vi "Image.vi"(8 "error in":errorcluster) -> (0 "error out":errorcluster)   [LabVIEW 2019, in "Image.lvlib"]
uses:
  Image.lvlib
  User Event/Controls/UE Abort Action.ctl
  LED/SubVI/Image Para.ctl
  MiControl-E/LV Source/ImageSystem/Cradle Zyla_1117/Ctl/seletion.ctl
  <vilib>/vision/Image Controls.llb/IMAQ Image.ctl
  <vilib>/Utility/error.llb/Error Cluster From Error Code.vi
  <vilib>/ErrorRing/Error Ring.xnode
  Queues/Queues.lvlib
  LED/LED.lvlib
  Motion/Allmotion/Allmotion.lvlib
  Camera/Andor/Andor.lvlib
  <vilib>/vision/NI_Vision_Development_Module.lvlib
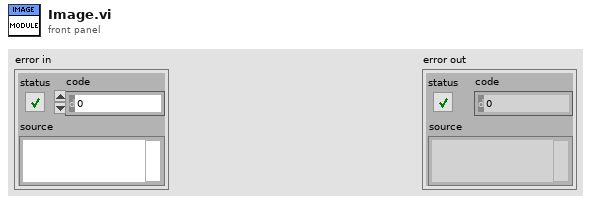
[diagram p1: front panel]
types:
  T1 = typedef "LED.lvlib/Image Para.ctl" = cluster{"Marker":T2, "Power(Amp)":u8, "set shutter(s)":dbl, "Cube":enum16{"1", "2", "3", "4", "5", "6", "7", "8"}}
  T2 = typedef "seletion.ctl" = enum16{"None", "Red", "Green", "Blue", "UV", "Green Laser", "Blue-Red", "UV-Red", "BF", "UV-IR"}
  T3 = typedef "IMAQ Image.ctl" = refnum<image>
  T4 = typedef "ROI Descriptor" = cluster{"Global Rectangle":i32[], "Contours":cluster{"ID":enum32{"External", "Internal"}, "Type":u32, "Coordinates":i32[]}[]}
  T5 = cluster{"Image Para":T1[], "Acquire Total":i32, "Acquire Count":i32, "Dichroic Position":string[], "Acquire Time":string, "Image Path":path, "Focus Positions":i32[], "Focus Total":i32, "Focus Count":i32, "Focus Score":sgl[], "Temp Image(U16)":T3, "Round Total":i32, "Round Count":i32, "Sharpest Position":i32, "Align Total":i32, "Align Count":i32, "Best Wheel Position":string, "Match Center":cluster{"x":sgl, "y":sgl}[], "Temp Image(U8)":T3, "Pattern Image(U8)":T3, "Match ROI":T4, "Max Score":dbl}
  T6 = typedef "UE Abort Action.ctl" = enum16{"Create", "Get", "Destroy"}
  T7 = cluster{"Image Path":path, "Start Offset":i32, "Template Path":path, "Disable Fine Search":bool, "ROI":T4}
  T8 = enum32{"Differentiation", "Gradient", "Prewitt", "Roberts", "Sigma", "Sobel"}
  T9 = cluster{"Number of Matches Requested":i32, "Minimum Match Score":sgl, "Angle Ranges":cluster{"Start Angle":sgl, "End Angle":sgl}[]}
  T10 = cluster{"um/pixel":dbl, "um/step":dbl, "Image Width":dbl, "Image Height":dbl}
  T11 = typedef "Image Type" = u32
  T12 = typedef "Image.lvlib/SEQ Data.ctl" = cluster{"Acquire Done?":bool, "Focus Done?":bool, "Align Done?":bool, "No Position Match?":bool, "Best Wheel Position":string, "Match Done?":bool, "Match Score":dbl, "Focus Score":dbl, "Match Position":cluster{"x":sgl, "y":sgl}, "Flower Position":i32[]}
  T13 = typedef "Rendezvous RefNum" = refnum<k1>
  T14 = typedef "Andor.lvlib/SEQ Data.ctl" = cluster{"Initialize Sucess?":bool, "Image Ref":T3, "VI Refnum":refnum<vi>}
  T15 = cluster{"Position":cluster{"x":sgl, "y":sgl}, "Angle":sgl, "Scale":sgl, "Score":sgl, "Bounding Box":cluster{"x":sgl, "y":sgl}[]}[]
  T16 = cluster{"Position":cluster{"x":sgl, "y":sgl}, "Angle":sgl, "Scale":sgl, "Score":sgl, "Bounding Box":cluster{"x":sgl, "y":sgl}[]}
  T17 = typedef "Allmotion.lvlib/SEQ Data.ctl" = cluster{"Position":i32[], "Arrived?":bool, "VISA name":refnum<visa-resource-name>, "Initialize Done?":bool, "State":string, "VI Refnum":refnum<vi>, "Dichroic Position":string[]}
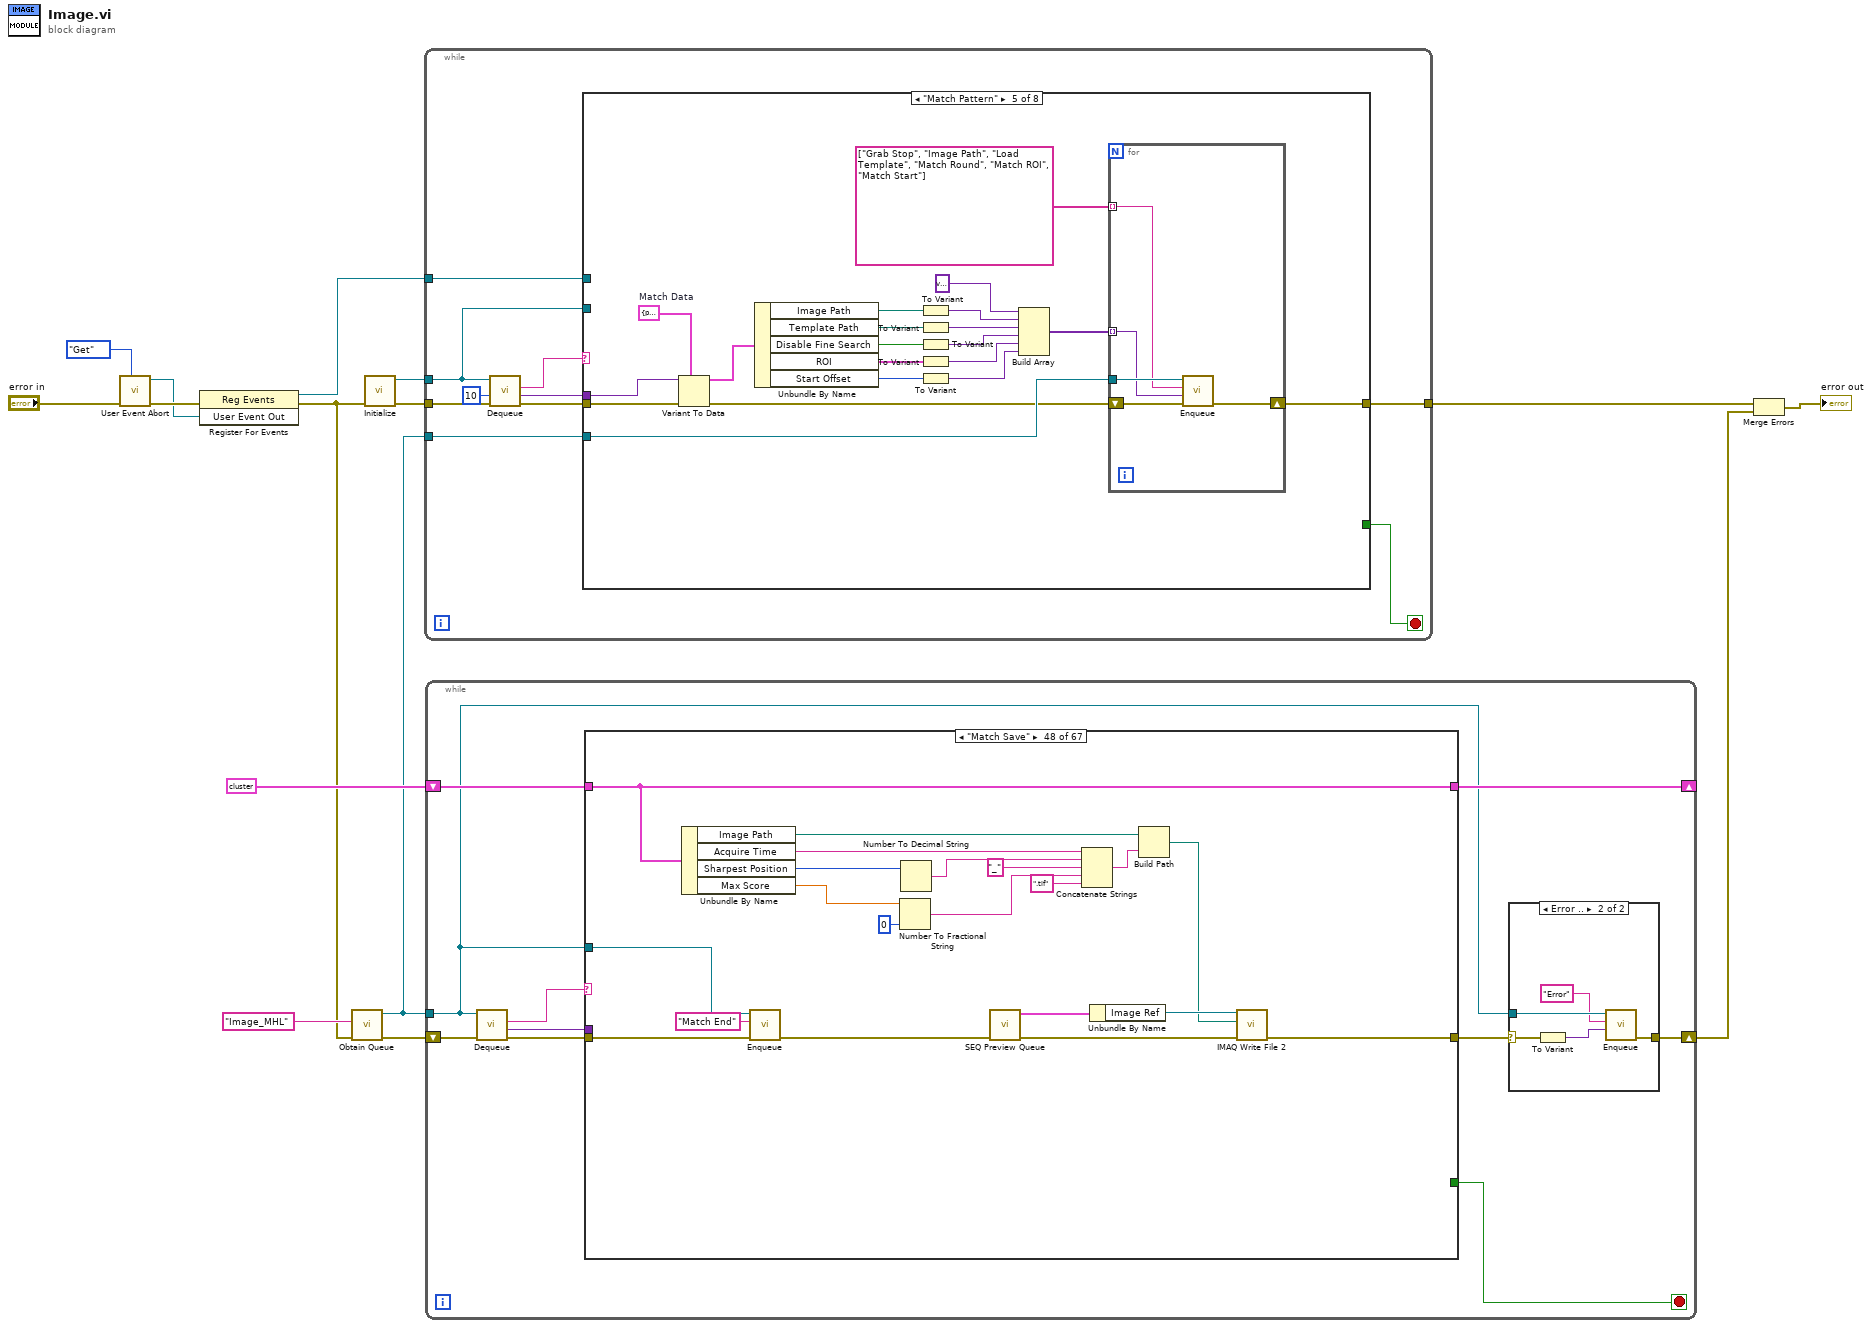
[diagram p0: block diagram]
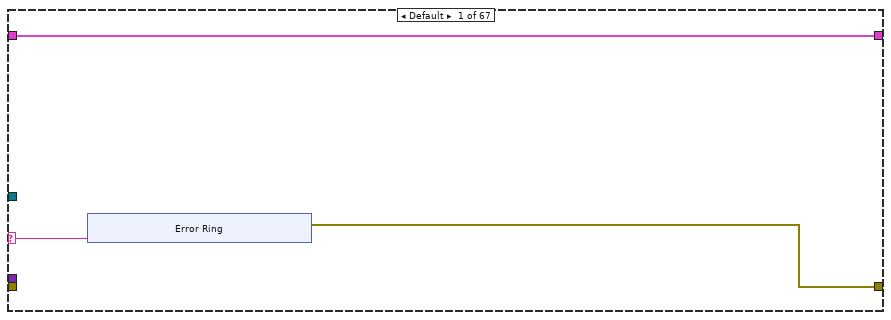
[diagram p2: hidden frame]
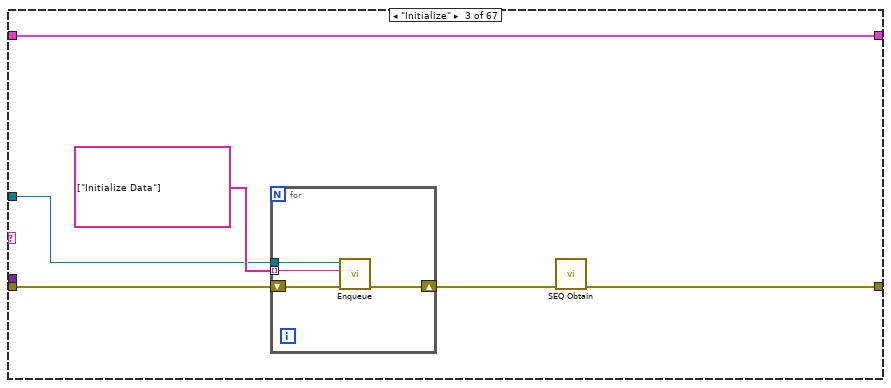
[diagram p4: hidden frame]
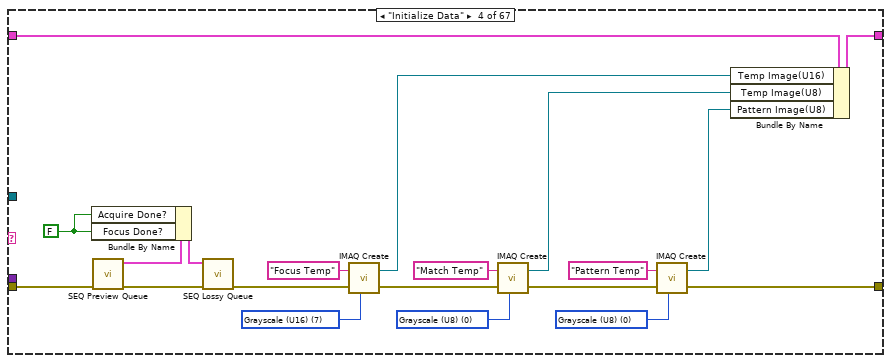
[diagram p5: hidden frame]
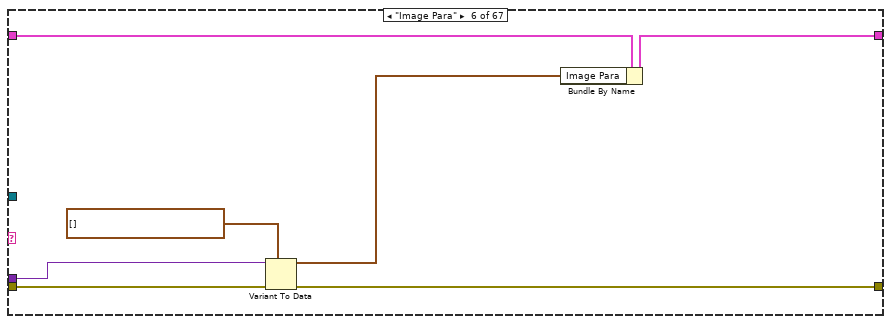
[diagram p7: hidden frame]
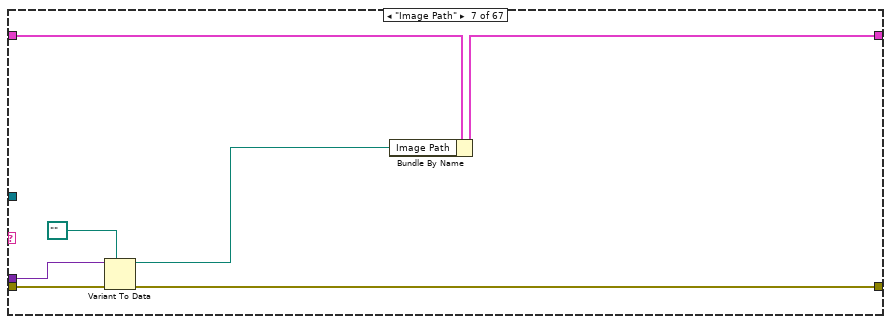
[diagram p8: hidden frame]
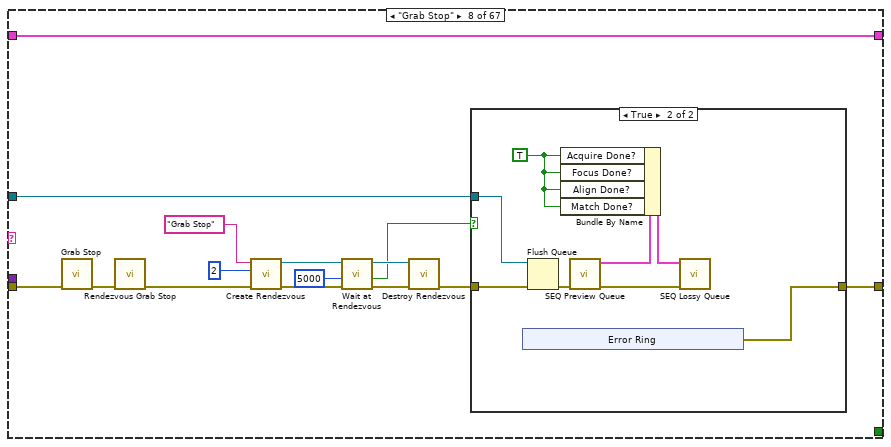
[diagram p9: hidden frame]
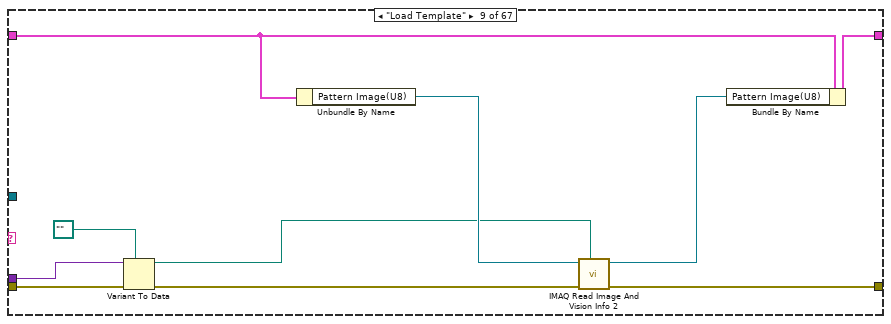
[diagram p11: hidden frame]
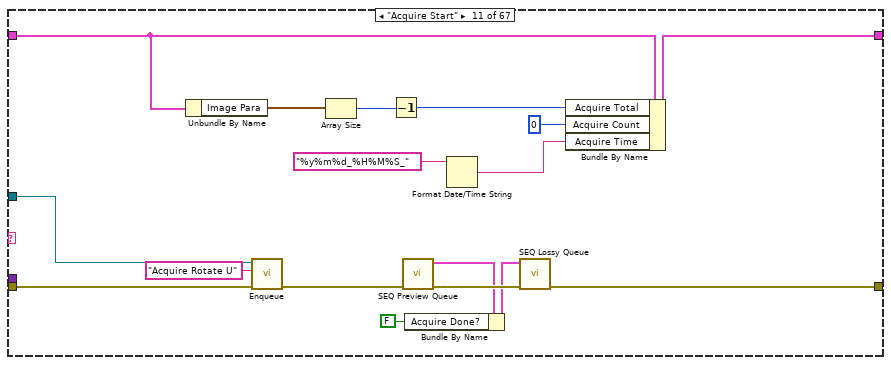
[diagram p13: hidden frame]
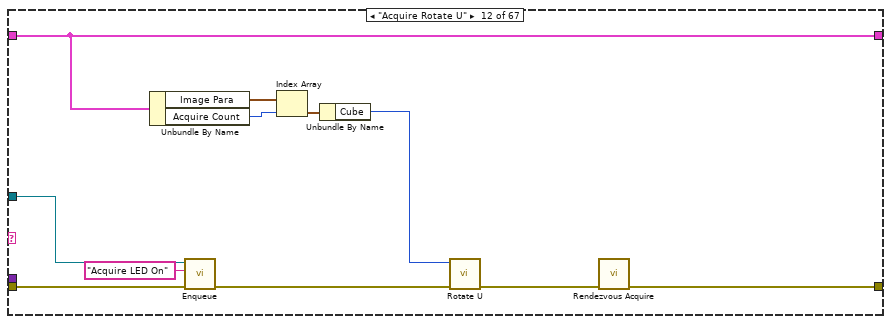
[diagram p14: hidden frame]
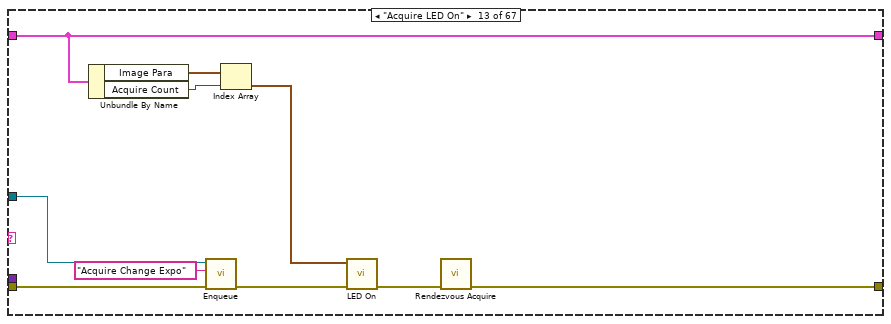
[diagram p15: hidden frame]
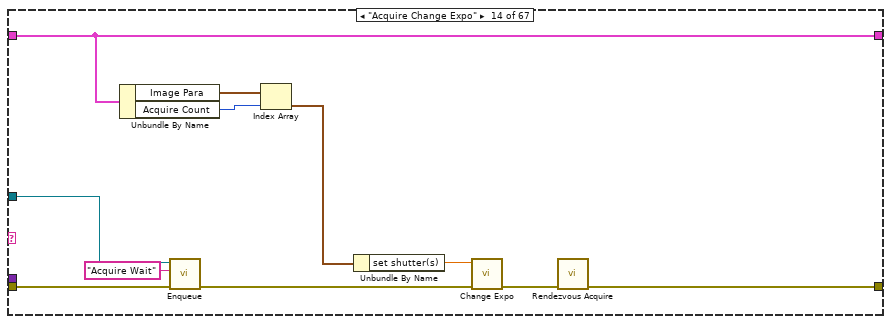
[diagram p16: hidden frame]
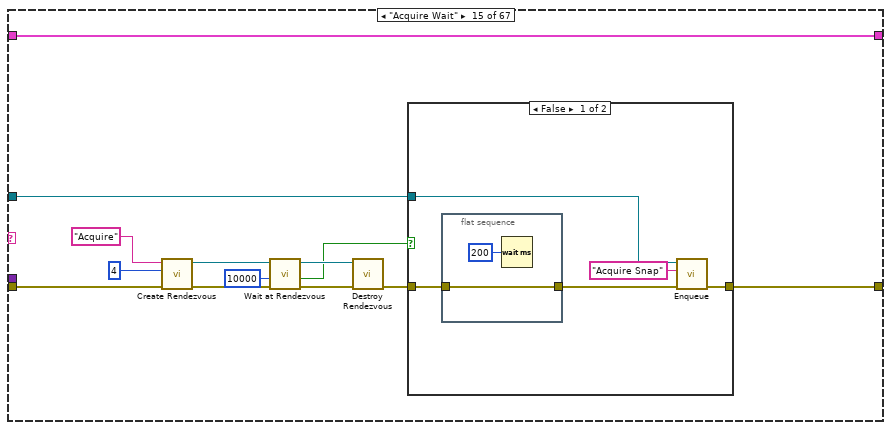
[diagram p17: hidden frame]
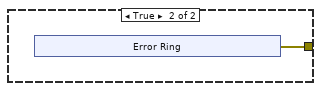
[diagram p18: hidden frame]
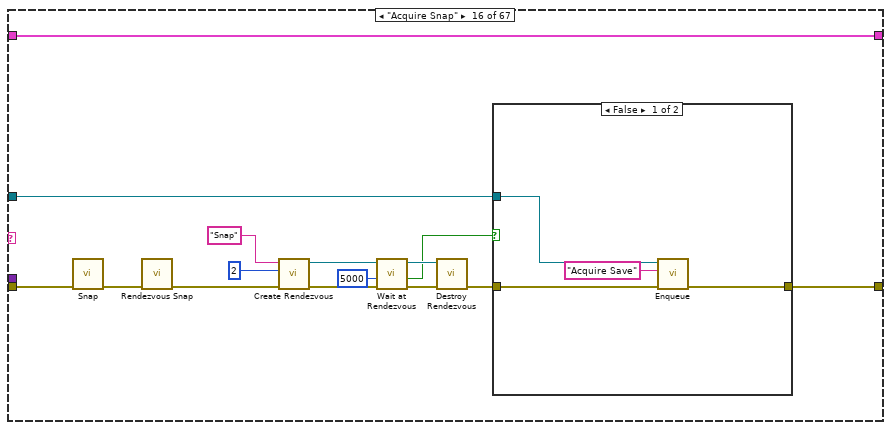
[diagram p19: hidden frame]
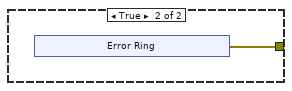
[diagram p20: hidden frame]
diagram:
  n1 = call "User Event Abort.vi"("Action"=UE_Abort_Action."Get", "Error In"="error in") -> ("Error Out"=w13:errorcluster, "User Event Out"=w12:refnum<user-event>)  [unwired: 8 in]
  n2 = register-events(error in=w13, w12) -> (reference out=w11:refnum<event-registration>, error out=w3:errorcluster)  [unwired: 1 in]
  n3 = call "Obtain Queue.vi"("Error In"=w3, "Queue Name"="Image_MHL") -> ("Error Out"=w9:errorcluster, "queue out"=w4:refnum<queue>)  [unwired: 8 in]
  n4 = call "Initialize.vi"("Error In"=w3) -> ("Error Out"=w2:errorcluster, "Queue out"=w1:refnum<queue>)  [unwired: 9 in]
  n5 = while {
    tunnel: w2 -> [w25]
    tunnel: w1 -> [w20]
    tunnel: [w19] -> w8
    tunnel: w11 -> [w18]
    tunnel: w4 -> [w16]
    stop <- w17 stop-if-true
    n6 = call "Dequeue.vi"("Error In"=w25, "timeout in ms (-1)"=10, "Queue in"=w20) -> ("Error Out"=w24:errorcluster, "Data"=w22:variant, "State"=w23:string)  [unwired: 5 in, 1 out]
    n7 = case shown="\"Match Pattern\"" w23 {
      selector: w23 -> [w26 _ _ _ _ _ _ _]
      tunnel: w24 -> [w29 w33 w47 w67 w92 w108 w120 w128]
      tunnel: w22 -> [_ _ w46 w66 w91 w107 _ _]
      tunnel: w20 -> [_ _ _ _ _ _ _ _]
      tunnel: [w29 w32 w51 w70 w95 w111 w119 w127] -> w19
      tunnel: w18 -> [_ _ _ _ _ _ _ w126]
      tunnel: [_ _ _ _ _ _ TRUE _] -> w17
      tunnel: w16 -> [_ w31 w50 w69 w94 w110 w118 _]
      frame "Typo", Default {
        n8 = Concatenate Strings("Typo: " ("string"), w26) -> (w28:string)
        n9 = One Button Dialog(message=w28) -> ()  [unwired: 1 in, 1 out]
      }
      frame "Initialize" {
        n10 = for {
          tunnel: w31 -> [w35]
          shift-right: [w36] -> w32
          shift-left: w33 -> [w37]
          tunnel: string[] ["Initialize"] -> [w34] mode=indexing
          n11 = call "Enqueue.vi"("Error In"=w37, "State"=w34, "Queue in"=w35) -> ("Error Out"=w36:errorcluster)  [unwired: 7 in, 1 out]
        }
      }
      frame "Acquire Image" {
        w45 = cluster{"Image Para":T1[], "Image Path":path} {"Image Para"=[], "Image Path"=path ""}  # Acquire Data
        w38 = variant
        n12 = Variant To Data(error in=w47, type=w45, Variant=w46) -> (data=w43:cluster{"Image Para":T1[], "Image Path":path}, error out=w44:errorcluster)
        n13 = Unbundle By Name(w43) -> ("Image Para"=w42:T1[], "Image Path"=w41:path)
        n14 = To Variant(anything=w42) -> (Variant=w40:variant)
        n15 = To Variant(anything=w41) -> (Variant=w39:variant)
        n16 = Build Array(w38, w40, w39, w38) -> (w49:variant[])
        n17 = for {
          tunnel: w50 -> [w55]
          shift-right: [w56] -> w51
          shift-left: w44 -> [w54]
          tunnel: w49 -> [w53] mode=indexing
          tunnel: string[] ["Grab Stop", "Image Para", "Image Path", "Acquire Start"] -> [w52] mode=indexing
          n18 = call "Enqueue.vi"("Error In"=w54, "Data"=w53, "State"=w52, "Queue in"=w55) -> ("Error Out"=w56:errorcluster)  [unwired: 6 in, 1 out]
        }
      }
      frame "Focus Search" {
        w62 = cluster{"Image Path":path, "Start Offset":i32} {"Image Path"=path "", "Start Offset"=0}  # Focus Data
        n19 = Variant To Data(error in=w67, type=w62, Variant=w66) -> (data=w61:cluster{"Image Path":path, "Start Offset":i32}, error out=w65:errorcluster)
        n20 = Unbundle By Name(w61) -> ("Image Path"=w60:path, "Start Offset"=w59:i32)
        n21 = To Variant(anything=w60) -> (Variant=w64:variant)
        n22 = To Variant(anything=w59) -> (Variant=w58:variant)
        n23 = Build Array(variant, w64, w58) -> (w63:variant[])
        n24 = for {
          tunnel: w69 -> [w74]
          shift-right: [w75] -> w70
          shift-left: w65 -> [w73]
          tunnel: string[] ["Grab Stop", "Image Path", "Focus Start"] -> [w72] mode=indexing
          tunnel: w63 -> [w71] mode=indexing
          n25 = call "Enqueue.vi"("Error In"=w73, "Data"=w71, "State"=w72, "Queue in"=w74) -> ("Error Out"=w75:errorcluster)  [unwired: 6 in, 1 out]
        }
      }
      frame "Match Pattern" {
        w79 = T7 {"Image Path"=path "", "Start Offset"=0, "Template Path"=path "", "Disable Fine Search"=FALSE, "ROI"={"Global Rectangle"=[], "Contours"=[]}}  # Match Data
        n26 = Variant To Data(error in=w92, type=w79, Variant=w91) -> (data=w87:T7, error out=w90:errorcluster)
        n27 = Unbundle By Name(w87) -> ("Image Path"=w86:path, "Template Path"=w83:path, "Disable Fine Search"=w82:bool, "ROI"=w77:T4, "Start Offset"=w78:i32)
        n28 = To Variant(anything=w86) -> (Variant=w89:variant)
        n29 = To Variant(anything=w83) -> (Variant=w85:variant)
        n30 = To Variant(anything=w82) -> (Variant=w81:variant)
        n31 = To Variant(anything=w77) -> (Variant=w80:variant)
        n32 = To Variant(anything=w78) -> (Variant=w76:variant)
        n33 = Build Array(variant, w89, w85, w81, w80, w76) -> (w88:variant[])
        n34 = for {
          tunnel: w94 -> [w99]
          shift-right: [w100] -> w95
          shift-left: w90 -> [w98]
          tunnel: string[] ["Grab Stop", "Image Path", "Load Template", "Match Round", "Match ROI", "Match Start"] -> [w97] mode=indexing
          tunnel: w88 -> [w96] mode=indexing
          n35 = call "Enqueue.vi"("Error In"=w98, "Data"=w96, "State"=w97, "Queue in"=w99) -> ("Error Out"=w100:errorcluster)  [unwired: 6 in, 1 out]
        }
      }
      frame "Align Laser" {
        w101 = variant
        n36 = Variant To Data(error in=w108, type=path "", Variant=w107) -> (data=w102:path, error out=w106:errorcluster)
        n37 = To Variant(anything=w102) -> (Variant=w105:variant)
        n38 = Build Array(w101, w105, w101) -> (w104:variant[])
        n39 = for {
          tunnel: w110 -> [w115]
          shift-right: [w116] -> w111
          shift-left: w106 -> [w114]
          tunnel: string[] ["Grab Stop", "Image Path", "Align Start"] -> [w113] mode=indexing
          tunnel: w104 -> [w112] mode=indexing
          n40 = call "Enqueue.vi"("Error In"=w114, "Data"=w112, "State"=w113, "Queue in"=w115) -> ("Error Out"=w116:errorcluster)  [unwired: 6 in, 1 out]
        }
      }
      frame "Close" {
        n41 = for {
          tunnel: w118 -> [w123]
          shift-right: [w124] -> w119
          shift-left: w120 -> [w125]
          tunnel: string[] ["Close"] -> [w122] mode=indexing
          n42 = call "Enqueue.vi"("Error In"=w125, "State"=w122, "Queue in"=w123) -> ("Error Out"=w124:errorcluster)  [unwired: 7 in, 1 out]
        }
      }
      frame "Idle" {
        n43 = event shown="[1] <User Event Out>: User Event" {
          selector: w126 -> [_ w134]
          dyn-events: _ -> [_ _]
          timeout: 10 -> [_ _]
          tunnel: w128 -> [w130 w132]
          tunnel: [w130 w133] -> w127
          event Timeout {
            n44 = event-data() -> ()  [unwired: 1 in, 3 out]
          }
          event User Event {
            n45 = event-data() -> ()  [unwired: 1 in, 4 out]
            n46 = call "Close.vi"("Error In"=w132) -> ("Error Out"=w131:errorcluster)  [unwired: 10 in]
            n47 = Unregister For Events(event registration refnum=w134, error in=w131) -> (error out=w133:errorcluster)
          }
        }
      }
    }
  }
  n48 = while {
    tunnel: w4 -> [w136]
    shift-right: [w139] -> _
    shift-left: T5 {"Image Para"=[], "Acquire Total"=0, "Acquire Count"=0, "Dichroic Position"=[], "Acquire Time"="", "Image Path"=path "", "Focus Positions"=[], "Focus Total"=0, "Focus Count"=0, "Focus Score"=[], "Temp Image(U16)"=refnum, "Round Total"=0, "Round Count"=0, "Sharpest Position"=0, "Align Total"=0, "Align Count"=0, "Best Wheel Position"="", "Match Center"=[], "Temp Image(U8)"=refnum, "Pattern Image(U8)"=refnum, "Match ROI"={"Global Rectangle"=[], "Contours"=[]}, "Max Score"=0.0} -> [w140]
    shift-right: [w138] -> w6
    shift-left: w9 -> [w144]
    stop <- w135 stop-if-true
    n49 = call "Dequeue.vi"("Error In"=w144, "Queue in"=w136) -> ("Error Out"=w141:errorcluster, "Data"=w142:variant, "State"=w143:string)  [unwired: 6 in, 1 out]
    n50 = case shown="\"Match Save\"" w143 {
      selector: w143 -> [w146 _ _ _ _ _ _ _ _ _ _ _ _ _ _ _ _ _ _ _ _ _ _ _ _ _ _ _ _ _ _ _ _ _ _ _ _ _ _ _ _ _ _ _ _ _ _ _ _ _ _ _ _ _ _ _ _ _ _ _ _ _ _ _ _ _ _]
      tunnel: w136 -> [_ _ w160 _ _ _ _ w204 _ _ w255 w270 w280 w291 w294 w319 w345 w367 _ _ w415 w430 w458 w484 w508 w526 w561 w582 w604 w607 w635 _ _ _ _ w694 w709 w737 w769 w794 w806 w824 w867 w898 w920 w946 w949 w982 _ _ w1018 w1038 w1070 w1094 w1120 w1135 w1155 w1181 w1211 w1235 w1262 _ _ _ _ w1298 w1314]
      tunnel: w142 -> [_ _ _ _ _ w193 w200 _ w234 _ _ _ _ _ _ _ _ _ _ _ w400 _ _ _ _ _ _ _ _ _ _ _ _ w666 w673 w680 _ _ _ _ _ _ _ _ _ _ _ _ _ _ _ _ _ _ _ _ _ _ _ _ _ _ _ w1290 _ _ _]
      tunnel: w141 -> [_ w155 w161 w186 w188 w194 w201 w216 w236 w242 w256 w271 w281 w292 w304 w332 w347 w371 w388 w396 w402 w441 w471 w486 w509 w539 w562 w583 w601 w620 w637 w651 w658 w667 w674 w682 w720 w750 w771 w795 w807 w837 w863 w899 w921 w943 w962 w984 w997 w1004 w1019 w1050 w1068 w1107 w1131 w1136 w1159 w1193 w1209 w1248 w1264 w1276 w1287 w1291 w1295 w1299 w1315]
      tunnel: w140 -> [w147 w156 w159 w182 w187 w195 w202 w217 w240 w243 w260 w269 w278 w288 w305 w333 w361 w373 w395 w397 w422 w447 w472 w500 w510 w544 w563 w578 w603 w621 w644 w657 w659 w669 w676 w701 w726 w751 w773 w799 w808 w842 w864 w900 w916 w944 w963 w990 w1003 w1005 w1033 w1052 w1066 w1108 w1127 w1140 w1160 w1195 w1207 w1249 w1271 w1285 w1286 w1288 w1294 w1296 w1311]
      tunnel: [w147 w156 w159 w178 w187 w191 w197 w217 w239 w243 w258 w269 w278 w288 w305 w333 w361 w366 w395 w397 w419 w447 w472 w489 w504 w524 w559 w587 w603 w621 w644 w657 w659 w668 w675 w698 w726 w751 w772 w797 w802 w822 w864 w896 w925 w934 w963 w990 w1003 w1005 w1024 w1052 w1066 w1108 w1127 w1133 w1153 w1195 w1207 w1249 w1271 w1285 w1286 w1288 w1294 w1296 w1311] -> w139
      tunnel: [w145 w155 w157 w169 w188 w189 w198 w203 w241 w242 w244 w264 w272 w284 w293 w320 w348 w370 w393 w396 w406 w429 w459 w487 w505 w525 w560 w580 w598 w608 w638 w655 w658 w663 w672 w686 w708 w738 w762 w781 w803 w823 w866 w897 w918 w935 w950 w985 w1001 w1004 w1013 w1037 w1069 w1095 w1121 w1134 w1154 w1180 w1210 w1236 w1265 w1283 w1287 errorcluster {"status"=FALSE, "code"=0, "source"=""} ("Error Out") w1295 w1297 w1307] -> w137
      tunnel: [_ _ _ _ _ _ _ _ _ _ _ _ _ _ _ _ _ _ _ _ _ _ _ _ _ _ _ _ _ _ _ _ _ _ _ _ _ _ _ _ _ _ _ _ _ _ _ _ _ _ _ _ _ _ _ _ _ _ _ _ _ _ _ _ _ _ TRUE] -> w135
      frame Default {
        n51 = xnode "Error Ring"("parameter 0"=w146) -> ("error out"=w145:errorcluster)
      }
      frame "------Initialize------" {
      }
      frame "Initialize" {
        n52 = for {
          tunnel: w160 -> [w164]
          shift-right: [w165] -> w158
          shift-left: w161 -> [w166]
          tunnel: string[] ["Initialize Data"] -> [w163] mode=indexing
          n53 = call "Enqueue.vi"("Error In"=w166, "State"=w163, "Queue in"=w164) -> ("Error Out"=w165:errorcluster)  [unwired: 7 in, 1 out]
        }
        n54 = call "SEQ Obtain.vi"("error in"=w158) -> ("error out"=w157:errorcluster)  [unwired: 9 in, 1 out]
      }
      frame "Initialize Data" {
        w173 = T11 0 items=["Grayscale (U8)", "Grayscale (I16)", "Grayscale (SGL)", "Complex (CSG)", "RGB (U32)", "HSL (U32)", "RGB (U64)", "Grayscale (U16)"] ("Image Type")
        w174 = T11 0 items=["Grayscale (U8)", "Grayscale (I16)", "Grayscale (SGL)", "Complex (CSG)", "RGB (U32)", "HSL (U32)", "RGB (U64)", "Grayscale (U16)"] ("Image Type")
        w180 = T11 7 items=["Grayscale (U8)", "Grayscale (I16)", "Grayscale (SGL)", "Complex (CSG)", "RGB (U32)", "HSL (U32)", "RGB (U64)", "Grayscale (U16)"] ("Image Type")
        w176 = FALSE ("Acquire Done?")
        n55 = call "SEQ Preview Queue.vi"("error in"=w186) -> ("error out"=w185:errorcluster, "SEQ Data"=w184:T12)  [unwired: 9 in]
        n56 = Bundle By Name(cluster=w184, "Acquire Done?"=w176, "Focus Done?"=w176) -> (w183:T12)
        n57 = call "SEQ Lossy Queue.vi"("error in"=w185, "SEQ Data"=w183) -> ("error out"=w181:errorcluster)  [unwired: 9 in]
        n58 = call "IMAQ Create"("Image Name"="Focus Temp", "Image Type"=w180, "error in (no error)"=w181) -> ("New Image"=w177:T3, "error out"=w171:errorcluster)  [unwired: 2 in]
        n59 = call "IMAQ Create"("Image Name"="Match Temp", "Image Type"=w174, "error in (no error)"=w171) -> ("New Image"=w168:T3, "error out"=w170:errorcluster)  [unwired: 2 in]
        n60 = call "IMAQ Create"("Image Name"="Pattern Temp", "Image Type"=w173, "error in (no error)"=w170) -> ("New Image"=w167:T3, "error out"=w169:errorcluster)  [unwired: 2 in]
        n61 = Bundle By Name(cluster=w182, "Temp Image(U16)"=w177, "Temp Image(U8)"=w168, "Pattern Image(U8)"=w167) -> (w178:T5)
      }
      frame "------Functions------" {
      }
      frame "Image Para" {
        n62 = Variant To Data(error in=w194, type=T1[] [], Variant=w193) -> (data=w190:T1[], error out=w189:errorcluster)
        n63 = Bundle By Name(cluster=w195, "Image Para"=w190) -> (w191:T5)
      }
      frame "Image Path" {
        n64 = Variant To Data(error in=w201, type=path "", Variant=w200) -> (data=w196:path, error out=w198:errorcluster)
        n65 = Bundle By Name(cluster=w202, "Image Path"=w196) -> (w197:T5)
      }
      frame "Grab Stop" {
        n66 = call "Grab Stop.vi"("Error In"=w216) -> ("Error Out"=w215:errorcluster)  [unwired: 10 in]
        n67 = call "Rendezvous Grab Stop.vi"("Error In"=w215) -> ("Error Out"=w207:errorcluster)  [unwired: 10 in]
        n68 = call <vilib>:"Create Rendezvous.vi"("error in (no error)"=w207, "size (2)"=2, "name (unnamed)"="Grab Stop") -> ("error out"=w214:errorcluster, "rendezvous"=w211:T13)  [unwired: 2 in, 1 out]
        n69 = call <vilib>:"Wait at Rendezvous.vi"("error in (no error)"=w214, "ms timeout (-1)"=5000, "rendezvous"=w211) -> ("error out"=w209:errorcluster, "timed out"=w205:bool, "rendezvous out"=w208:T13)  [unwired: 2 in]
        n70 = call <vilib>:"Destroy Rendezvous.vi"("error in (no error)"=w209, "rendezvous"=w208) -> ("error out"=w206:errorcluster)  [unwired: 4 in, 1 out]
        n71 = case shown="True" w205 {
          tunnel: w206 -> [w218 w226]
          tunnel: w204 -> [_ w225]
          tunnel: [w218 w220] -> w203
          frame False {
          }
          frame True {
            w219 = TRUE ("Acquire Done?")
            n72 = xnode "Error Ring"() -> ("error out"=w220:errorcluster)
            n73 = Flush Queue(queue=w225, error in (no error)=w226) -> (error out=w224:errorcluster)  [unwired: 2 out]
            n74 = call "SEQ Preview Queue.vi"("error in"=w224) -> ("error out"=w223:errorcluster, "SEQ Data"=w222:T12)  [unwired: 9 in]
            n75 = Bundle By Name(cluster=w222, "Acquire Done?"=w219, "Focus Done?"=w219, "Align Done?"=w219, "Match Done?"=w219) -> (w221:T12)
            n76 = call "SEQ Lossy Queue.vi"("error in"=w223, "SEQ Data"=w221) -> ()  [unwired: 9 in, 1 out]
          }
        }
      }
      frame "Load Template" {
        n77 = Variant To Data(error in=w236, type=path "", Variant=w234) -> (data=w232:path, error out=w235:errorcluster)
        n78 = Unbundle By Name(w240) -> ("Pattern Image(U8)"=w237:T3)
        n79 = call "IMAQ Read Image And Vision Info 2"("File Path"=w232, "error in (no error)"=w235, "Image"=w237) -> ("error out"=w241:errorcluster, "Image Out"=w238:T3)  [unwired: 6 in, 1 out]
        n80 = Bundle By Name(cluster=w240, "Pattern Image(U8)"=w238) -> (w239:T5)
      }
      frame "------Acquire Image------" {
      }
      frame "Acquire Start" {
        n81 = Unbundle By Name(w260) -> ("Image Para"=w259:T1[])
        n82 = call "Enqueue.vi"("Error In"=w256, "State"="Acquire Rotate U", "Queue in"=w255) -> ("Error Out"=w249:errorcluster)  [unwired: 7 in, 1 out]
        n83 = Array Size(array=w259) -> (size(s)=w253:i32)
        n84 = Decrement(x=w253) -> (x-1=w252:i32)
        n85 = call "SEQ Preview Queue.vi"("error in"=w249) -> ("error out"=w248:errorcluster, "SEQ Data"=w247:T12)  [unwired: 9 in]
        n86 = Bundle By Name(cluster=w247, "Acquire Done?"=FALSE) -> (w246:T12)
        n87 = Format Date/Time String(time format string (%c)="%y%m%d_%H%M%S_") -> (date/time string=w250:string)  [unwired: 2 in]
        n88 = call "SEQ Lossy Queue.vi"("error in"=w248, "SEQ Data"=w246) -> ("error out"=w244:errorcluster)  [unwired: 9 in]
        n89 = Bundle By Name(cluster=w260, "Acquire Total"=w252, "Acquire Count"=0, "Acquire Time"=w250) -> (w258:T5)
      }
      frame "Acquire Rotate U" {
        n90 = Unbundle By Name(w269) -> ("Image Para"=w268:T1[], "Acquire Count"=w267:i32)
        n91 = call "Enqueue.vi"("Error In"=w271, "State"="Acquire LED On", "Queue in"=w270) -> ("Error Out"=w263:errorcluster)  [unwired: 7 in, 1 out]
        n92 = Index Array(array=w268, index=w267) -> (element=w266:T1)
        n93 = Unbundle By Name(w266) -> ("Cube"=w261:enum16{"1", "2", "3", "4", "5", "6", "7", "8"})
        n94 = call "Rotate U.vi"("Error In"=w263, "Cube"=w261) -> ("Error Out"=w262:errorcluster)  [unwired: 9 in]
        n95 = call "Rendezvous Acquire.vi"("Error In"=w262) -> ("Error Out"=w264:errorcluster)  [unwired: 10 in]
      }
      frame "Acquire LED On" {
        n96 = Unbundle By Name(w278) -> ("Image Para"=w277:T1[], "Acquire Count"=w276:i32)
        n97 = call "Enqueue.vi"("Error In"=w281, "State"="Acquire Change Expo", "Queue in"=w280) -> ("Error Out"=w275:errorcluster)  [unwired: 7 in, 1 out]
        n98 = Index Array(array=w277, index=w276) -> (element=w274:T1)
        n99 = call "LED On.vi"("Error In"=w275, "Image Para"=w274) -> ("Error Out"=w273:errorcluster)  [unwired: 9 in]
        n100 = call "Rendezvous Acquire.vi"("Error In"=w273) -> ("Error Out"=w272:errorcluster)  [unwired: 10 in]
      }
      frame "Acquire Change Expo" {
        n101 = Unbundle By Name(w288) -> ("Image Para"=w287:T1[], "Acquire Count"=w286:i32)
        n102 = call "Enqueue.vi"("Error In"=w292, "State"="Acquire Wait", "Queue in"=w291) -> ("Error Out"=w289:errorcluster)  [unwired: 7 in, 1 out]
        n103 = Index Array(array=w287, index=w286) -> (element=w283:T1)
        n104 = Unbundle By Name(w283) -> ("set shutter(s)"=w282:dbl)
        n105 = call "Change Expo.vi"("Error In"=w289, "Expo(s)"=w282) -> ("Error Out"=w285:errorcluster)  [unwired: 9 in]
        n106 = call "Rendezvous Acquire.vi"("Error In"=w285) -> ("Error Out"=w284:errorcluster)  [unwired: 10 in]
      }
      frame "Acquire Wait" {
        n107 = call <vilib>:"Create Rendezvous.vi"("error in (no error)"=w304, "size (2)"=4, "name (unnamed)"="Acquire") -> ("error out"=w303:errorcluster, "rendezvous"=w301:T13)  [unwired: 2 in, 1 out]
        n108 = call <vilib>:"Wait at Rendezvous.vi"("error in (no error)"=w303, "ms timeout (-1)"=10000, "rendezvous"=w301) -> ("error out"=w302:errorcluster, "timed out"=w296:bool, "rendezvous out"=w300:T13)  [unwired: 2 in]
        n109 = call <vilib>:"Destroy Rendezvous.vi"("error in (no error)"=w302, "rendezvous"=w300) -> ("error out"=w295:errorcluster)  [unwired: 4 in, 1 out]
        n110 = case shown="False" w296 {
          tunnel: w295 -> [w307 _]
          tunnel: w294 -> [w310 _]
          tunnel: [w308 w313] -> w293
          frame False {
            n111 = flat-sequence {
              tunnel: w307 -> [w311]
              tunnel: [w311] -> w306
              frame #0 {
                n112 = Wait (ms)(milliseconds to wait=u32 200) -> ()  [unwired: 1 out]
              }
            }
            n113 = call "Enqueue.vi"("Error In"=w306, "State"="Acquire Snap", "Queue in"=w310) -> ("Error Out"=w308:errorcluster)  [unwired: 7 in, 1 out]
          }
          frame True {
            n114 = xnode "Error Ring"() -> ("error out"=w313:errorcluster)
          }
        }
      }
      frame "Acquire Snap" {
        n115 = call "Snap.vi"("Error In"=w332) -> ("Error Out"=w331:errorcluster)  [unwired: 10 in]
        n116 = call "Rendezvous Snap.vi"("Error In"=w331) -> ("Error Out"=w330:errorcluster)  [unwired: 10 in]
        n117 = call <vilib>:"Create Rendezvous.vi"("error in (no error)"=w330, "size (2)"=2, "name (unnamed)"="Snap") -> ("error out"=w329:errorcluster, "rendezvous"=w327:T13)  [unwired: 2 in, 1 out]
        n118 = call <vilib>:"Wait at Rendezvous.vi"("error in (no error)"=w329, "ms timeout (-1)"=5000, "rendezvous"=w327) -> ("error out"=w328:errorcluster, "timed out"=w321:bool, "rendezvous out"=w326:T13)  [unwired: 2 in]
        n119 = call <vilib>:"Destroy Rendezvous.vi"("error in (no error)"=w328, "rendezvous"=w326) -> ("error out"=w322:errorcluster)  [unwired: 4 in, 1 out]
        n120 = case shown="False" w321 {
          tunnel: w322 -> [w337 _]
          tunnel: [w336 w338] -> w320
          tunnel: w319 -> [w335 _]
          frame False {
            n121 = call "Enqueue.vi"("Error In"=w337, "State"="Acquire Save", "Queue in"=w335) -> ("Error Out"=w336:errorcluster)  [unwired: 7 in, 1 out]
          }
          frame True {
            n122 = xnode "Error Ring"() -> ("error out"=w338:errorcluster)
          }
        }
      }
      frame "Acquire Save" {
        n123 = Unbundle By Name(w361) -> ("Image Path"=w351:path, "Acquire Time"=w354:string, "Image Para"=w360:T1[], "Acquire Count"=w359:i32)
        n124 = call "Enqueue.vi"("Error In"=w347, "State"="Acquire Next", "Queue in"=w345) -> ("Error Out"=w346:errorcluster)  [unwired: 7 in, 1 out]
        n125 = Index Array(array=w360, index=w359) -> (element=w355:T1)
        n126 = Unbundle By Name(w355) -> ("Marker"=w358:T2, "Cube"=w356:enum16{"1", "2", "3", "4", "5", "6", "7", "8"})
        n127 = Format Into String(format string="%s_%s", w358, w356) -> (resulting string=w353:string)  [unwired: 2 in, 1 out]
        n128 = call "SEQ Preview Queue.vi"("error in"=w346) -> ("error out"=w363:errorcluster, "SEQ Data"=w364:T14)  [unwired: 9 in]
        n129 = Concatenate Strings(w354, w353, ".tif" ("string")) -> (w350:string)
        n130 = Unbundle By Name(w364) -> ("Image Ref"=w362:T3)
        n131 = Build Path(base path=w351, name or relative path=w350) -> (appended path=w349:path)
        n132 = call-poly "IMAQ Write File 2"("error in (no error)"=w363, "File Path"=w349, "Image"=w362) -> ("error out"=w348:errorcluster)  [unwired: 7 in, 1 out]
      }
      frame "Acquire Next" {
        n133 = Unbundle By Name(w373) -> ("Acquire Total"=w372:i32, "Acquire Count"=w368:i32)
        n134 = Equal?(x=w372, y=w368) -> (x = y?=w369:bool)
        n135 = case shown="True" w369 {
          tunnel: w371 -> [w379 w384]
          tunnel: [w378 w383] -> w370
          tunnel: w368 -> [w375 _]
          tunnel: w367 -> [w377 w382]
          tunnel: [w374 0] -> w365
          frame False {
            n136 = Increment(x=w375) -> (x+1=w374:i32)
            n137 = call "Enqueue.vi"("Error In"=w379, "State"="Acquire Rotate U", "Queue in"=w377) -> ("Error Out"=w378:errorcluster)  [unwired: 7 in, 1 out]
          }
          frame True {
            n138 = call "Enqueue.vi"("Error In"=w384, "State"="Acquire End", "Queue in"=w382) -> ("Error Out"=w383:errorcluster)  [unwired: 7 in, 1 out]
          }
        }
        n139 = Bundle By Name(cluster=w373, "Acquire Count"=w365) -> (w366:T5)
      }
      frame "Acquire End" {
        n140 = call "Change Expo.vi"("Error In"=w388, "Expo(s)"=0.05) -> ("Error Out"=w387:errorcluster)  [unwired: 9 in]
        n141 = call "Grab.vi"("Error In"=w387) -> ("Error Out"=w386:errorcluster)  [unwired: 10 in]
        n142 = call "LED Off.vi"("Error In"=w386) -> ("Error Out"=w389:errorcluster)  [unwired: 10 in]
        n143 = call "SEQ Preview Queue.vi"("error in"=w389) -> ("error out"=w394:errorcluster, "SEQ Data"=w392:T12)  [unwired: 9 in]
        n144 = Bundle By Name(cluster=w392, "Acquire Done?"=TRUE) -> (w391:T12)
        n145 = call "SEQ Lossy Queue.vi"("error in"=w394, "SEQ Data"=w391) -> ("error out"=w393:errorcluster)  [unwired: 9 in]
      }
      frame "------Focus Search------" {
      }
      frame "Focus Start" {
        w420 = 65  # Interation
        w421 = -100  # Interval
        w399 = 0  # Start Step
        n146 = Variant To Data(error in=w402, type=w399, Variant=w400) -> (data=w398:i32, error out=w401:errorcluster)
        n147 = call "Enqueue.vi"("Error In"=w401, "State"="Focus Move", "Queue in"=w415) -> ("Error Out"=w408:errorcluster)  [unwired: 7 in, 1 out]
        n148 = for {
          N: w420 -> [_]
          tunnel: w398 -> [w426]
          tunnel: w421 -> [w427]
          tunnel: [w424] -> w418 mode=indexing
          i -> [w423]
          n149 = Multiply(x=w427, y=w423) -> (x*y=w425:i32)
          n150 = Add(x=w426, y=w425) -> (x+y=w424:i32)
        }
        n151 = Decrement(x=w420) -> (x-1=w417:i32)
        n152 = Format Date/Time String(time format string (%c)="%y%m%d_%H%M%S_") -> (date/time string=w409:string)  [unwired: 2 in]
        n153 = call "SEQ Preview Queue.vi"("error in"=w408) -> ("error out"=w407:errorcluster, "SEQ Data"=w405:T12)  [unwired: 9 in]
        n154 = Bundle By Name(cluster=w405, "Focus Done?"=FALSE) -> (w404:T12)
        n155 = Bundle By Name(cluster=w422, "Round Total"=1, "Round Count"=0, "Focus Positions"=w418, "Focus Total"=w417, "Focus Count"=0, "Focus Score"=sgl[] [] ("Detection Score"), "Acquire Time"=w409) -> (w419:T5)
        n156 = call "SEQ Lossy Queue.vi"("error in"=w407, "SEQ Data"=w404) -> ("error out"=w406:errorcluster)  [unwired: 9 in]
      }
      frame "Focus Move" {
        n157 = Unbundle By Name(w447) -> ("Focus Positions"=w446:i32[], "Focus Count"=w445:i32)
        n158 = Index Array(array=w446, index=w445) -> (element=w444:i32)
        n159 = Number To Decimal String(number=w444) -> (decimal integer string=w443:string)  [unwired: 1 in]
        n160 = call "Move Axis 3.vi"("Error In"=w441, "Position"=w443) -> ("Error Out"=w442:errorcluster)  [unwired: 9 in]
        n161 = call "Rendezvous Focus.vi"("Error In"=w442) -> ("Error Out"=w440:errorcluster)  [unwired: 10 in]
        n162 = xnode "Error Ring"() -> ("error out"=w428:errorcluster)
        n163 = call <vilib>:"Create Rendezvous.vi"("error in (no error)"=w440, "size (2)"=2, "name (unnamed)"="Focus") -> ("error out"=w439:errorcluster, "rendezvous"=w436:T13)  [unwired: 2 in, 1 out]
        n164 = call <vilib>:"Wait at Rendezvous.vi"("error in (no error)"=w439, "ms timeout (-1)"=10000, "rendezvous"=w436) -> ("error out"=w438:errorcluster, "timed out"=w431:bool, "rendezvous out"=w437:T13)  [unwired: 2 in]
        n165 = call <vilib>:"Destroy Rendezvous.vi"("error in (no error)"=w438, "rendezvous"=w437) -> ("error out"=w432:errorcluster)  [unwired: 4 in, 1 out]
        n166 = case shown="False" w431 {
          tunnel: w432 -> [w455 _]
          tunnel: w430 -> [w453 _]
          tunnel: [w454 w457] -> w429
          tunnel: w428 -> [_ w457]
          frame False {
            n167 = call "Enqueue.vi"("Error In"=w455, "State"="Focus Snap", "Queue in"=w453) -> ("Error Out"=w454:errorcluster)  [unwired: 7 in, 1 out]
          }
          frame True {
          }
        }
      }
      frame "Focus Snap" {
        n168 = call "Snap.vi"("Error In"=w471) -> ("Error Out"=w470:errorcluster)  [unwired: 10 in]
        n169 = call "Rendezvous Snap.vi"("Error In"=w470) -> ("Error Out"=w469:errorcluster)  [unwired: 10 in]
        n170 = call <vilib>:"Create Rendezvous.vi"("error in (no error)"=w469, "size (2)"=2, "name (unnamed)"="Snap") -> ("error out"=w468:errorcluster, "rendezvous"=w466:T13)  [unwired: 2 in, 1 out]
        n171 = call <vilib>:"Wait at Rendezvous.vi"("error in (no error)"=w468, "ms timeout (-1)"=5000, "rendezvous"=w466) -> ("error out"=w467:errorcluster, "timed out"=w460:bool, "rendezvous out"=w465:T13)  [unwired: 2 in]
        n172 = call <vilib>:"Destroy Rendezvous.vi"("error in (no error)"=w467, "rendezvous"=w465) -> ("error out"=w461:errorcluster)  [unwired: 4 in, 1 out]
        n173 = case shown="False" w460 {
          tunnel: w461 -> [w476 _]
          tunnel: [w475 w477] -> w459
          tunnel: w458 -> [w474 _]
          frame False {
            n174 = call "Enqueue.vi"("Error In"=w476, "State"="Focus Detection", "Queue in"=w474) -> ("Error Out"=w475:errorcluster)  [unwired: 7 in, 1 out]
          }
          frame True {
            n175 = xnode "Error Ring"() -> ("error out"=w477:errorcluster)
          }
        }
      }
      frame "Focus Detection" {
        n176 = call "Enqueue.vi"("Error In"=w486, "State"="Focus Next", "Queue in"=w484) -> ("Error Out"=w485:errorcluster)  [unwired: 7 in, 1 out]
        n177 = call "SEQ Preview Queue.vi"("error in"=w485) -> ("error out"=w498:errorcluster, "SEQ Data"=w501:T14)  [unwired: 9 in]
        n178 = Unbundle By Name(w500) -> ("Focus Score"=w491:sgl[], "Temp Image(U16)"=w497:T3)
        n179 = Unbundle By Name(w501) -> ("Image Ref"=w499:T3)
        n180 = call "IMAQ EdgeDetection"("Method"=T8."Sobel", "error in (no error)"=w498, "Image Dst"=w497, "Image Src"=w499) -> ("error out"=w495:errorcluster, "Image Dst Out"=w494:T3)  [unwired: 6 in]
        n181 = call "IMAQ Histograph"("error in (no error)"=w495, "Image"=w494) -> ("error out"=w487:errorcluster, "Standard  Deviation"=w492:sgl, "Mean Value"=w493:sgl)  [unwired: 6 in, 1 out]
        n182 = Divide(x=w492, y=w493) -> (x/y=w490:sgl)
        n183 = Build Array (concatenate)(w491, w490) -> (w488:sgl[])
        n184 = Bundle By Name(cluster=w500, "Focus Score"=w488) -> (w489:T5)
      }
      frame "Focus Next" {
        n185 = Unbundle By Name(w510) -> ("Focus Total"=w507:i32, "Focus Count"=w506:i32)
        n186 = Equal?(x=w507, y=w506) -> (x = y?=w502:bool)
        n187 = case shown="True" w502 {
          tunnel: w509 -> [w514 w521]
          tunnel: w508 -> [w513 w520]
          tunnel: w506 -> [w516 _]
          tunnel: [w515 0] -> w503
          tunnel: [w511 w518] -> w505
          frame False {
            n188 = Increment(x=w516) -> (x+1=w515:i32)
            n189 = call "Enqueue.vi"("Error In"=w514, "State"="Focus Move", "Queue in"=w513) -> ("Error Out"=w511:errorcluster)  [unwired: 7 in, 1 out]
          }
          frame True {
            n190 = call "Enqueue.vi"("Error In"=w521, "State"="Focus Change", "Queue in"=w520) -> ("Error Out"=w518:errorcluster)  [unwired: 7 in, 1 out]
          }
        }
        n191 = Bundle By Name(cluster=w510, "Focus Count"=w503) -> (w504:T5)
      }
      frame "Focus Change" {
        n192 = Unbundle By Name(w544) -> ("Focus Positions"=w541:i32[], "Focus Score"=w543:sgl[])
        n193 = To Double Precision Float(number=w543) -> (double precision float=w542:dbl[])
        n194 = Array Max & Min(array=w542) -> (max index (indices)=w540:i32)  [unwired: 3 out]
        n195 = Index Array(array=w541, index=w540) -> (element=w523:i32)
        n196 = Number To Decimal String(number=w523) -> (decimal integer string=w538:string)  [unwired: 1 in]
        n197 = call "Move Axis 3.vi"("Error In"=w539, "Position"=w538) -> ("Error Out"=w537:errorcluster)  [unwired: 9 in]
        n198 = xnode "Error Ring"() -> ("error out"=w522:errorcluster)
        n199 = call "Rendezvous Focus.vi"("Error In"=w537) -> ("Error Out"=w536:errorcluster)  [unwired: 10 in]
        n200 = Bundle By Name(cluster=w544, "Sharpest Position"=w523) -> (w524:T5)
        n201 = call <vilib>:"Create Rendezvous.vi"("error in (no error)"=w536, "size (2)"=2, "name (unnamed)"="Focus") -> ("error out"=w532:errorcluster, "rendezvous"=w533:T13)  [unwired: 2 in, 1 out]
        n202 = call <vilib>:"Wait at Rendezvous.vi"("error in (no error)"=w532, "ms timeout (-1)"=10000, "rendezvous"=w533) -> ("error out"=w530:errorcluster, "timed out"=w527:bool, "rendezvous out"=w529:T13)  [unwired: 2 in]
        n203 = call <vilib>:"Destroy Rendezvous.vi"("error in (no error)"=w530, "rendezvous"=w529) -> ("error out"=w528:errorcluster)  [unwired: 4 in, 1 out]
        n204 = case shown="False" w527 {
          tunnel: w528 -> [w553 _]
          tunnel: w526 -> [w551 _]
          tunnel: [w552 w554] -> w525
          tunnel: w522 -> [_ w554]
          frame False {
            n205 = call "Enqueue.vi"("Error In"=w553, "State"="Focus Switch", "Queue in"=w551) -> ("Error Out"=w552:errorcluster)  [unwired: 7 in, 1 out]
          }
          frame True {
          }
        }
      }
      frame "Focus Switch" {
        n206 = Unbundle By Name(w563) -> ("Round Total"=w558:i32, "Round Count"=w556:i32)
        n207 = Equal?(x=w558, y=w556) -> (x = y?=w557:bool)
        n208 = case shown="True" w557 {
          tunnel: w562 -> [w567 w574]
          tunnel: w561 -> [w565 w573]
          tunnel: [w566 w572] -> w560
          tunnel: w556 -> [w569 _]
          tunnel: [w568 0] -> w555
          frame False {
            n209 = Increment(x=w569) -> (x+1=w568:i32)
            n210 = call "Enqueue.vi"("Error In"=w567, "State"="Focus Start Fine", "Queue in"=w565) -> ("Error Out"=w566:errorcluster)  [unwired: 7 in, 1 out]
          }
          frame True {
            n211 = call "Enqueue.vi"("Error In"=w574, "State"="Focus Analysis", "Queue in"=w573) -> ("Error Out"=w572:errorcluster)  [unwired: 7 in, 1 out]
          }
        }
        n212 = Bundle By Name(cluster=w563, "Round Count"=w555) -> (w559:T5)
      }
      frame "Focus Start Fine" {
        w575 = 100  # Fine Offset
        w588 = 9  # Interation
        w589 = -25  # Interval
        n213 = Unbundle By Name(w578) -> ("Sharpest Position"=w577:i32)
        n214 = call "Enqueue.vi"("Error In"=w583, "State"="Focus Move", "Queue in"=w582) -> ("Error Out"=w580:errorcluster)  [unwired: 7 in, 1 out]
        n215 = Add(x=w577, y=w575) -> (x+y=w576:i32)
        n216 = for {
          N: w588 -> [_]
          tunnel: w576 -> [w593]
          tunnel: w589 -> [w594]
          tunnel: [w591] -> w586 mode=indexing
          i -> [w590]
          n217 = Multiply(x=w594, y=w590) -> (x*y=w592:i32)
          n218 = Add(x=w593, y=w592) -> (x+y=w591:i32)
        }
        n219 = Decrement(x=w588) -> (x-1=w585:i32)
        n220 = Bundle By Name(cluster=w578, "Focus Positions"=w586, "Focus Total"=w585, "Focus Count"=0, "Focus Score"=sgl[] [] ("Detection Score")) -> (w587:T5)
      }
      frame "Focus Analysis" {
        n221 = Unbundle By Name(w603) -> ("Focus Score"=w606:sgl[])
        n222 = call "Enqueue.vi"("Error In"=w601, "State"="Focus Snap Final", "Queue in"=w604) -> ("Error Out"=w600:errorcluster)  [unwired: 7 in, 1 out]
        n223 = To Double Precision Float(number=w606) -> (double precision float=w605:dbl[])
        n224 = Array Max & Min(array=w605) -> (max value=w595:dbl)  [unwired: 3 out]
        n225 = call "SEQ Preview Queue.vi"("error in"=w600) -> ("error out"=w599:errorcluster, "SEQ Data"=w597:T12)  [unwired: 9 in]
        n226 = Bundle By Name(cluster=w597, "Focus Score"=w595) -> (w596:T12)
        n227 = call "SEQ Lossy Queue.vi"("error in"=w599, "SEQ Data"=w596) -> ("error out"=w598:errorcluster)  [unwired: 9 in]
      }
      frame "Focus Snap Final" {
        n228 = call "Snap.vi"("Error In"=w620) -> ("Error Out"=w619:errorcluster)  [unwired: 10 in]
        n229 = call "Rendezvous Snap.vi"("Error In"=w619) -> ("Error Out"=w618:errorcluster)  [unwired: 10 in]
        n230 = call <vilib>:"Create Rendezvous.vi"("error in (no error)"=w618, "size (2)"=2, "name (unnamed)"="Snap") -> ("error out"=w617:errorcluster, "rendezvous"=w615:T13)  [unwired: 2 in, 1 out]
        n231 = call <vilib>:"Wait at Rendezvous.vi"("error in (no error)"=w617, "ms timeout (-1)"=5000, "rendezvous"=w615) -> ("error out"=w616:errorcluster, "timed out"=w609:bool, "rendezvous out"=w614:T13)  [unwired: 2 in]
        n232 = call <vilib>:"Destroy Rendezvous.vi"("error in (no error)"=w616, "rendezvous"=w614) -> ("error out"=w610:errorcluster)  [unwired: 4 in, 1 out]
        n233 = case shown="False" w609 {
          tunnel: w610 -> [w625 _]
          tunnel: [w624 w626] -> w608
          tunnel: w607 -> [w623 _]
          frame False {
            n234 = call "Enqueue.vi"("Error In"=w625, "State"="Focus Save", "Queue in"=w623) -> ("Error Out"=w624:errorcluster)  [unwired: 7 in, 1 out]
          }
          frame True {
            n235 = xnode "Error Ring"() -> ("error out"=w626:errorcluster)
          }
        }
      }
      frame "Focus Save" {
        n236 = Unbundle By Name(w644) -> ("Image Path"=w641:path, "Acquire Time"=w643:string, "Sharpest Position"=w633:i32)
        n237 = call "Enqueue.vi"("Error In"=w637, "State"="Focus End", "Queue in"=w635) -> ("Error Out"=w636:errorcluster)  [unwired: 7 in, 1 out]
        n238 = Number To Decimal String(number=w633) -> (decimal integer string=w632:string)  [unwired: 1 in]
        n239 = call "SEQ Preview Queue.vi"("error in"=w636) -> ("error out"=w646:errorcluster, "SEQ Data"=w647:T14)  [unwired: 9 in]
        n240 = Concatenate Strings(w643, w632, ".tif" ("string")) -> (w640:string)
        n241 = Unbundle By Name(w647) -> ("Image Ref"=w645:T3)
        n242 = Build Path(base path=w641, name or relative path=w640) -> (appended path=w639:path)
        n243 = call-poly "IMAQ Write File 2"("error in (no error)"=w646, "File Path"=w639, "Image"=w645) -> ("error out"=w638:errorcluster)  [unwired: 7 in, 1 out]
      }
      frame "Focus End" {
        n244 = call "Change Expo.vi"("Error In"=w651, "Expo(s)"=0.05) -> ("Error Out"=w650:errorcluster)  [unwired: 9 in]
        n245 = call "Grab.vi"("Error In"=w650) -> ("Error Out"=w649:errorcluster)  [unwired: 10 in]
        n246 = call "SEQ Preview Queue.vi"("error in"=w649) -> ("error out"=w656:errorcluster, "SEQ Data"=w654:T12)  [unwired: 9 in]
        n247 = Bundle By Name(cluster=w654, "Focus Done?"=TRUE) -> (w653:T12)
        n248 = call "SEQ Lossy Queue.vi"("error in"=w656, "SEQ Data"=w653) -> ("error out"=w655:errorcluster)  [unwired: 9 in]
      }
      frame "------Match Pattern------" {
      }
      frame "Match Round" {
        w665 = FALSE  # Disable Fine Search
        n249 = Variant To Data(error in=w667, type=w665, Variant=w666) -> (data=w664:bool, error out=w663:errorcluster)
        n250 = Select(t=1 ("Round Count"), s=w664, f=0 ("Round Count")) -> (s? t:f=w660:i32)
        n251 = Bundle By Name(cluster=w669, "Round Count"=w660) -> (w668:T5)
      }
      frame "Match ROI" {
        n252 = Variant To Data(error in=w674, type=T4 {"Global Rectangle"=[], "Contours"=[]} ("Match ROI"), Variant=w673) -> (data=w670:T4, error out=w672:errorcluster)
        n253 = Bundle By Name(cluster=w676, "Match ROI"=w670) -> (w675:T5)
      }
      frame "Match Start" {
        w699 = 65  # Interation
        w700 = -100  # Interval
        w679 = 0  # Start Step
        n254 = Variant To Data(error in=w682, type=w679, Variant=w680) -> (data=w678:i32, error out=w681:errorcluster)
        n255 = call "Enqueue.vi"("Error In"=w681, "State"="Match Move", "Queue in"=w694) -> ("Error Out"=w688:errorcluster)  [unwired: 7 in, 1 out]
        n256 = for {
          N: w699 -> [_]
          tunnel: w678 -> [w705]
          tunnel: w700 -> [w706]
          tunnel: [w703] -> w697 mode=indexing
          i -> [w702]
          n257 = Multiply(x=w706, y=w702) -> (x*y=w704:i32)
          n258 = Add(x=w705, y=w704) -> (x+y=w703:i32)
        }
        n259 = Decrement(x=w699) -> (x-1=w696:i32)
        n260 = Format Date/Time String(time format string (%c)="%y%m%d_%H%M%S_") -> (date/time string=w689:string)  [unwired: 2 in]
        n261 = call "SEQ Preview Queue.vi"("error in"=w688) -> ("error out"=w687:errorcluster, "SEQ Data"=w685:T12)  [unwired: 9 in]
        n262 = Bundle By Name(cluster=w685, "Match Done?"=FALSE ("Focus Done?")) -> (w684:T12)
        n263 = Bundle By Name(cluster=w701, "Round Total"=1, "Focus Positions"=w697, "Focus Total"=w696, "Focus Count"=0, "Focus Score"=sgl[] [] ("Detection Score"), "Acquire Time"=w689, "Match Center"=cluster{"x":sgl, "y":sgl}[] []) -> (w698:T5)
        n264 = call "SEQ Lossy Queue.vi"("error in"=w687, "SEQ Data"=w684) -> ("error out"=w686:errorcluster)  [unwired: 9 in]
      }
      frame "Match Move" {
        n265 = Unbundle By Name(w726) -> ("Focus Positions"=w725:i32[], "Focus Count"=w724:i32)
        n266 = Index Array(array=w725, index=w724) -> (element=w723:i32)
        n267 = Number To Decimal String(number=w723) -> (decimal integer string=w722:string)  [unwired: 1 in]
        n268 = call "Move Axis 3.vi"("Error In"=w720, "Position"=w722) -> ("Error Out"=w721:errorcluster)  [unwired: 9 in]
        n269 = call "Rendezvous Focus.vi"("Error In"=w721) -> ("Error Out"=w719:errorcluster)  [unwired: 10 in]
        n270 = xnode "Error Ring"() -> ("error out"=w707:errorcluster)
        n271 = call <vilib>:"Create Rendezvous.vi"("error in (no error)"=w719, "size (2)"=2, "name (unnamed)"="Focus") -> ("error out"=w718:errorcluster, "rendezvous"=w715:T13)  [unwired: 2 in, 1 out]
        n272 = call <vilib>:"Wait at Rendezvous.vi"("error in (no error)"=w718, "ms timeout (-1)"=10000, "rendezvous"=w715) -> ("error out"=w717:errorcluster, "timed out"=w710:bool, "rendezvous out"=w716:T13)  [unwired: 2 in]
        n273 = call <vilib>:"Destroy Rendezvous.vi"("error in (no error)"=w717, "rendezvous"=w716) -> ("error out"=w711:errorcluster)  [unwired: 4 in, 1 out]
        n274 = case shown="False" w710 {
          tunnel: w711 -> [w734 _]
          tunnel: w709 -> [w732 _]
          tunnel: [w733 w736] -> w708
          tunnel: w707 -> [_ w736]
          frame False {
            n275 = call "Enqueue.vi"("Error In"=w734, "State"="Match Snap", "Queue in"=w732) -> ("Error Out"=w733:errorcluster)  [unwired: 7 in, 1 out]
          }
          frame True {
          }
        }
      }
      frame "Match Snap" {
        n276 = call "Snap.vi"("Error In"=w750) -> ("Error Out"=w749:errorcluster)  [unwired: 10 in]
        n277 = call "Rendezvous Snap.vi"("Error In"=w749) -> ("Error Out"=w748:errorcluster)  [unwired: 10 in]
        n278 = call <vilib>:"Create Rendezvous.vi"("error in (no error)"=w748, "size (2)"=2, "name (unnamed)"="Snap") -> ("error out"=w747:errorcluster, "rendezvous"=w745:T13)  [unwired: 2 in, 1 out]
        n279 = call <vilib>:"Wait at Rendezvous.vi"("error in (no error)"=w747, "ms timeout (-1)"=5000, "rendezvous"=w745) -> ("error out"=w746:errorcluster, "timed out"=w739:bool, "rendezvous out"=w744:T13)  [unwired: 2 in]
        n280 = call <vilib>:"Destroy Rendezvous.vi"("error in (no error)"=w746, "rendezvous"=w744) -> ("error out"=w740:errorcluster)  [unwired: 4 in, 1 out]
        n281 = case shown="False" w739 {
          tunnel: w740 -> [w755 _]
          tunnel: [w754 w756] -> w738
          tunnel: w737 -> [w753 _]
          frame False {
            n282 = call "Enqueue.vi"("Error In"=w755, "State"="Match Convert", "Queue in"=w753) -> ("Error Out"=w754:errorcluster)  [unwired: 7 in, 1 out]
          }
          frame True {
            n283 = xnode "Error Ring"() -> ("error out"=w756:errorcluster)
          }
        }
      }
      frame "Match Convert" {
        w766 = T11 0 items=["Grayscale (U8)", "Grayscale (I16)", "Grayscale (SGL)", "Complex (CSG)", "RGB (U32)", "HSL (U32)", "RGB (U64)", "Grayscale (U16)"] ("Image Type")
        n284 = call "Enqueue.vi"("Error In"=w771, "State"="Match Detection", "Queue in"=w769) -> ("Error Out"=w770:errorcluster)  [unwired: 7 in, 1 out]
        n285 = call "SEQ Preview Queue.vi"("error in"=w770) -> ("error out"=w767:errorcluster, "SEQ Data"=w774:T14)  [unwired: 9 in]
        n286 = Unbundle By Name(w773) -> ("Temp Image(U8)"=w764:T3)
        n287 = Unbundle By Name(w774) -> ("Image Ref"=w765:T3)
        n288 = call "IMAQ Cast Image 2"("Image Src"=w765, "Image Dst"=w764, "Image Type"=w766, "error in (no error)"=w767) -> ("Image Dst Out"=w763:T3, "error out"=w762:errorcluster)  [unwired: 10 in]
        n289 = Bundle By Name(cluster=w773, "Temp Image(U8)"=w763) -> (w772:T5)
      }
      frame "Match Detection" {
        w790 = 1 items=["All", "Low Discrepancy Sampling", "Grayscale Value Pyramid", "Gradients Pyramid"] ("Algorithm")
        n290 = Unbundle By Name(w799) -> ("Focus Score"=w798:sgl[], "Temp Image(U8)"=w787:T3, "Pattern Image(U8)"=w786:T3, "Match Center"=w784:cluster{"x":sgl, "y":sgl}[], "Match ROI"=w776:T4)
        n291 = call "Enqueue.vi"("Error In"=w795, "State"="Match Next", "Queue in"=w794) -> ("Error Out"=w788:errorcluster)  [unwired: 7 in, 1 out]
        n292 = call "IMAQ Match Pattern 4"("Image"=w787, "Algorithm"=w790, "Template Image"=w786, "ROI Descriptor"=w776, "Parameters"=T9 {"Number of Matches Requested"=1, "Minimum Match Score"=1.0, "Angle Ranges"=[]}, "error in (no error)"=w788, "Advanced Options"=cluster{"Item":u16, "Value":dbl}[] [{"Item"=0, "Value"=10.0}, {"Item"=2, "Value"=2.0}, {"Item"=5, "Value"=300.0}, {"Item"=6, "Value"=3.0}, {"Item"=7, "Value"=5.0}, {"Item"=8, "Value"=2.0}, {"Item"=1, "Value"=1.0}, {"Item"=3, "Value"=20.0}, {"Item"=4, "Value"=0.0}]) -> ("Matches (pixel)"=w792:T15, "error out"=w783:errorcluster)  [unwired: 4 in, 3 out]
        n293 = Index Array(array=w792) -> (element=w791:T16)  [unwired: 1 in]
        n294 = Unbundle By Name(w791) -> ("Score"=w778:sgl, "Position"=w777:cluster{"x":sgl, "y":sgl})
        n295 = call "SEQ Preview Queue.vi"("error in"=w783) -> ("error out"=w782:errorcluster, "SEQ Data"=w780:T12)  [unwired: 9 in]
        n296 = Build Array (concatenate)(w798, w778) -> (w796:sgl[])
        n297 = Build Array (concatenate)(w784, w777) -> (w785:cluster{"x":sgl, "y":sgl}[])
        n298 = Bundle By Name(cluster=w780, "Match Score"=w778) -> (w779:T12)
        n299 = Bundle By Name(cluster=w799, "Focus Score"=w796, "Match Center"=w785) -> (w797:T5)
        n300 = call "SEQ Lossy Queue.vi"("error in"=w782, "SEQ Data"=w779) -> ("error out"=w781:errorcluster)  [unwired: 9 in]
      }
      frame "Match Next" {
        n301 = Unbundle By Name(w808) -> ("Focus Total"=w805:i32, "Focus Count"=w804:i32)
        n302 = Equal?(x=w805, y=w804) -> (x = y?=w800:bool)
        n303 = case shown="True" w800 {
          tunnel: w807 -> [w812 w819]
          tunnel: w806 -> [w811 w818]
          tunnel: w804 -> [w814 _]
          tunnel: [w813 0] -> w801
          tunnel: [w809 w816] -> w803
          frame False {
            n304 = Increment(x=w814) -> (x+1=w813:i32)
            n305 = call "Enqueue.vi"("Error In"=w812, "State"="Match Move", "Queue in"=w811) -> ("Error Out"=w809:errorcluster)  [unwired: 7 in, 1 out]
          }
          frame True {
            n306 = call "Enqueue.vi"("Error In"=w819, "State"="Match Change", "Queue in"=w818) -> ("Error Out"=w816:errorcluster)  [unwired: 7 in, 1 out]
          }
        }
        n307 = Bundle By Name(cluster=w808, "Focus Count"=w801) -> (w802:T5)
      }
      frame "Match Change" {
        n308 = Unbundle By Name(w842) -> ("Focus Positions"=w839:i32[], "Focus Score"=w841:sgl[])
        n309 = To Double Precision Float(number=w841) -> (double precision float=w840:dbl[])
        n310 = Array Max & Min(array=w840) -> (max index (indices)=w838:i32)  [unwired: 3 out]
        n311 = Index Array(array=w839, index=w838) -> (element=w821:i32)
        n312 = Number To Decimal String(number=w821) -> (decimal integer string=w836:string)  [unwired: 1 in]
        n313 = Bundle By Name(cluster=w842, "Sharpest Position"=w821) -> (w822:T5)
        n314 = call "Move Axis 3.vi"("Error In"=w837, "Position"=w836) -> ("Error Out"=w835:errorcluster)  [unwired: 9 in]
        n315 = xnode "Error Ring"() -> ("error out"=w820:errorcluster)
        n316 = call "Rendezvous Focus.vi"("Error In"=w835) -> ("Error Out"=w834:errorcluster)  [unwired: 10 in]
        n317 = call <vilib>:"Create Rendezvous.vi"("error in (no error)"=w834, "size (2)"=2, "name (unnamed)"="Focus") -> ("error out"=w830:errorcluster, "rendezvous"=w831:T13)  [unwired: 2 in, 1 out]
        n318 = call <vilib>:"Wait at Rendezvous.vi"("error in (no error)"=w830, "ms timeout (-1)"=10000, "rendezvous"=w831) -> ("error out"=w828:errorcluster, "timed out"=w825:bool, "rendezvous out"=w827:T13)  [unwired: 2 in]
        n319 = call <vilib>:"Destroy Rendezvous.vi"("error in (no error)"=w828, "rendezvous"=w827) -> ("error out"=w826:errorcluster)  [unwired: 4 in, 1 out]
        n320 = case shown="False" w825 {
          tunnel: w826 -> [w851 _]
          tunnel: w824 -> [w849 _]
          tunnel: [w850 w852] -> w823
          tunnel: w820 -> [_ w852]
          frame False {
            n321 = call "Enqueue.vi"("Error In"=w851, "State"="Match Navigate", "Queue in"=w849) -> ("Error Out"=w850:errorcluster)  [unwired: 7 in, 1 out]
          }
          frame True {
          }
        }
      }
      frame "Match Navigate" {
        n322 = Unbundle By Name(w864) -> ("Match Center"=w879:cluster{"x":sgl, "y":sgl}[], "Focus Score"=w881:sgl[])
        n323 = call "SEQ Preview Queue.vi"("error in"=w863) -> ("error out"=w859:errorcluster, "SEQ Data"=w862:T17)  [unwired: 9 in]
        n324 = Unbundle By Name(w862) -> ("Position"=w861:i32[])
        n325 = To Double Precision Float(number=w881) -> (double precision float=w880:dbl[])
        n326 = To Double Precision Float(number=w861) -> (double precision float=w860:dbl[])
        n327 = Array Max & Min(array=w880) -> (max index (indices)=w878:i32)  [unwired: 3 out]
        n328 = Index Array(array=w879, index=w878) -> (element=w853:cluster{"x":sgl, "y":sgl})
        n329 = call "Align Position Convert.vi"("error in"=w859, "Resolution"=T10 {"um/pixel"=0.325, "um/step"=0.625, "Image Width"=2560.0, "Image Height"=2160.0}, "Focus Center"=w853, "Position in"=w860) -> ("error out"=w857:errorcluster, "Position out"=w858:dbl[])  [unwired: 6 in]
        n330 = To Long Integer(number=w858) -> (32bit integer=w855:i32[])
        n331 = call "Move.vi"("Error In"=w857, "Target Position"=w855) -> ("Error Out"=w856:errorcluster)  [unwired: 9 in]
        n332 = xnode "Error Ring"() -> ("error out"=w865:errorcluster)
        n333 = call "Rendezvous Focus.vi"("Error In"=w856) -> ("Error Out"=w877:errorcluster)  [unwired: 10 in]
        n334 = call <vilib>:"Create Rendezvous.vi"("error in (no error)"=w877, "size (2)"=2, "name (unnamed)"="Focus") -> ("error out"=w873:errorcluster, "rendezvous"=w874:T13)  [unwired: 2 in, 1 out]
        n335 = call <vilib>:"Wait at Rendezvous.vi"("error in (no error)"=w873, "ms timeout (-1)"=10000, "rendezvous"=w874) -> ("error out"=w871:errorcluster, "timed out"=w868:bool, "rendezvous out"=w870:T13)  [unwired: 2 in]
        n336 = call <vilib>:"Destroy Rendezvous.vi"("error in (no error)"=w871, "rendezvous"=w870) -> ("error out"=w869:errorcluster)  [unwired: 4 in, 1 out]
        n337 = case shown="False" w868 {
          tunnel: w869 -> [w890 _]
          tunnel: w867 -> [w888 _]
          tunnel: [w889 w891] -> w866
          tunnel: w865 -> [_ w891]
          frame False {
            n338 = call "Enqueue.vi"("Error In"=w890, "State"="Match Switch", "Queue in"=w888) -> ("Error Out"=w889:errorcluster)  [unwired: 7 in, 1 out]
          }
          frame True {
          }
        }
      }
      frame "Match Switch" {
        n339 = Unbundle By Name(w900) -> ("Round Total"=w895:i32, "Round Count"=w893:i32)
        n340 = Equal?(x=w895, y=w893) -> (x = y?=w894:bool)
        n341 = case shown="True" w894 {
          tunnel: w899 -> [w904 w911]
          tunnel: w898 -> [w902 w910]
          tunnel: [w903 w909] -> w897
          tunnel: w893 -> [w906 _]
          tunnel: [w905 0] -> w892
          frame False {
            n342 = Increment(x=w906) -> (x+1=w905:i32)
            n343 = call "Enqueue.vi"("Error In"=w904, "State"="Match Start Fine", "Queue in"=w902) -> ("Error Out"=w903:errorcluster)  [unwired: 7 in, 1 out]
          }
          frame True {
            n344 = call "Enqueue.vi"("Error In"=w911, "State"="Match Analysis", "Queue in"=w910) -> ("Error Out"=w909:errorcluster)  [unwired: 7 in, 1 out]
          }
        }
        n345 = Bundle By Name(cluster=w900, "Round Count"=w892) -> (w896:T5)
      }
      frame "Match Start Fine" {
        w913 = 100  # Fine Offset
        w926 = 9  # Interation
        w927 = -25  # Interval
        n346 = Unbundle By Name(w916) -> ("Sharpest Position"=w915:i32)
        n347 = call "Enqueue.vi"("Error In"=w921, "State"="Match Move", "Queue in"=w920) -> ("Error Out"=w918:errorcluster)  [unwired: 7 in, 1 out]
        n348 = Add(x=w915, y=w913) -> (x+y=w914:i32)
        n349 = for {
          N: w926 -> [_]
          tunnel: w914 -> [w931]
          tunnel: w927 -> [w932]
          tunnel: [w929] -> w924 mode=indexing
          i -> [w928]
          n350 = Multiply(x=w932, y=w928) -> (x*y=w930:i32)
          n351 = Add(x=w931, y=w930) -> (x+y=w929:i32)
        }
        n352 = Decrement(x=w926) -> (x-1=w923:i32)
        n353 = Bundle By Name(cluster=w916, "Focus Positions"=w924, "Focus Total"=w923, "Focus Count"=0, "Focus Score"=sgl[] [] ("Detection Score"), "Match Center"=cluster{"x":sgl, "y":sgl}[] []) -> (w925:T5)
      }
      frame "Match Analysis" {
        n354 = Unbundle By Name(w944) -> ("Focus Score"=w948:sgl[])
        n355 = call "Enqueue.vi"("Error In"=w943, "State"="Match Snap Final", "Queue in"=w946) -> ("Error Out"=w938:errorcluster)  [unwired: 7 in, 1 out]
        n356 = To Double Precision Float(number=w948) -> (double precision float=w947:dbl[])
        n357 = Array Max & Min(array=w947) -> (max value=w933:dbl)  [unwired: 3 out]
        n358 = call "SEQ Preview Queue.vi"("error in"=w938) -> ("error out"=w937:errorcluster, "SEQ Data"=w939:T17)  [unwired: 9 in]
        n359 = Unbundle By Name(w939) -> ("Position"=w936:i32[])
        n360 = call "SEQ Preview Queue.vi"("error in"=w937) -> ("error out"=w942:errorcluster, "SEQ Data"=w941:T12)  [unwired: 9 in]
        n361 = Bundle By Name(cluster=w941, "Match Score"=w933, "Flower Position"=w936) -> (w940:T12)
        n362 = call "SEQ Lossy Queue.vi"("error in"=w942, "SEQ Data"=w940) -> ("error out"=w935:errorcluster)  [unwired: 9 in]
        n363 = Bundle By Name(cluster=w944, "Max Score"=w933) -> (w934:T5)
      }
      frame "Match Snap Final" {
        n364 = call "Snap.vi"("Error In"=w962) -> ("Error Out"=w961:errorcluster)  [unwired: 10 in]
        n365 = call "Rendezvous Snap.vi"("Error In"=w961) -> ("Error Out"=w960:errorcluster)  [unwired: 10 in]
        n366 = call <vilib>:"Create Rendezvous.vi"("error in (no error)"=w960, "size (2)"=2, "name (unnamed)"="Snap") -> ("error out"=w959:errorcluster, "rendezvous"=w957:T13)  [unwired: 2 in, 1 out]
        n367 = call <vilib>:"Wait at Rendezvous.vi"("error in (no error)"=w959, "ms timeout (-1)"=5000, "rendezvous"=w957) -> ("error out"=w958:errorcluster, "timed out"=w951:bool, "rendezvous out"=w956:T13)  [unwired: 2 in]
        n368 = call <vilib>:"Destroy Rendezvous.vi"("error in (no error)"=w958, "rendezvous"=w956) -> ("error out"=w952:errorcluster)  [unwired: 4 in, 1 out]
        n369 = case shown="False" w951 {
          tunnel: w952 -> [w967 _]
          tunnel: [w966 w968] -> w950
          tunnel: w949 -> [w965 _]
          frame False {
            n370 = call "Enqueue.vi"("Error In"=w967, "State"="Match Save", "Queue in"=w965) -> ("Error Out"=w966:errorcluster)  [unwired: 7 in, 1 out]
          }
          frame True {
            n371 = xnode "Error Ring"() -> ("error out"=w968:errorcluster)
          }
        }
      }
      frame "Match Save" {
        n372 = Unbundle By Name(w990) -> ("Image Path"=w988:path, "Acquire Time"=w989:string, "Sharpest Position"=w980:i32, "Max Score"=w977:dbl)
        n373 = call "Enqueue.vi"("Error In"=w984, "State"="Match End", "Queue in"=w982) -> ("Error Out"=w983:errorcluster)  [unwired: 7 in, 1 out]
        n374 = Number To Fractional String(number=w977, precision (6)=i16 0) -> (F-format string=w975:string)  [unwired: 2 in]
        n375 = Number To Decimal String(number=w980) -> (decimal integer string=w979:string)  [unwired: 1 in]
        n376 = call "SEQ Preview Queue.vi"("error in"=w983) -> ("error out"=w992:errorcluster, "SEQ Data"=w993:T14)  [unwired: 9 in]
        n377 = Concatenate Strings(w989, w979, "_", w975, ".tif" ("string")) -> (w987:string)
        n378 = Unbundle By Name(w993) -> ("Image Ref"=w991:T3)
        n379 = Build Path(base path=w988, name or relative path=w987) -> (appended path=w986:path)
        n380 = call-poly "IMAQ Write File 2"("error in (no error)"=w992, "File Path"=w986, "Image"=w991) -> ("error out"=w985:errorcluster)  [unwired: 7 in, 1 out]
      }
      frame "Match End" {
        n381 = call "Change Expo.vi"("Error In"=w997, "Expo(s)"=0.05) -> ("Error Out"=w996:errorcluster)  [unwired: 9 in]
        n382 = call "Grab.vi"("Error In"=w996) -> ("Error Out"=w995:errorcluster)  [unwired: 10 in]
        n383 = call "SEQ Preview Queue.vi"("error in"=w995) -> ("error out"=w1002:errorcluster, "SEQ Data"=w1000:T12)  [unwired: 9 in]
        n384 = Bundle By Name(cluster=w1000, "Match Done?"=TRUE ("Focus Done?")) -> (w999:T12)
        n385 = call "SEQ Lossy Queue.vi"("error in"=w1002, "SEQ Data"=w999) -> ("error out"=w1001:errorcluster)  [unwired: 9 in]
      }
      frame "------Align Laser------" {
      }
      frame "Align Start" {
        n386 = call "Enqueue.vi"("Error In"=w1019, "State"="Align Rotate 6", "Queue in"=w1018) -> ("Error Out"=w1007:errorcluster)  [unwired: 7 in, 1 out]
        n387 = call "SEQ Preview Queue.vi"("error in"=w1007) -> ("SEQ Data"=w1032:T17)  [unwired: 9 in, 1 out]
        n388 = Unbundle By Name(w1032) -> ("Dichroic Position"=w1031:string[])
        n389 = Index Array(array=w1031) -> (element=w1025:string)  [unwired: 1 in]
        n390 = Fract/Exp String To Number(string=w1025) -> (number=w1029:dbl)  [unwired: 3 in, 1 out]
        n391 = call "Overlay Enable.vi"("Error In"=w1007) -> ("Error Out"=w1006:errorcluster)  [unwired: 10 in]
        n392 = Add(x=3.0, y=w1029) -> (x+y=w1026:dbl)
        n393 = for {
          N: 7 -> [_]
          tunnel: w1026 -> [w1036]
          tunnel: [w1034] -> w1028 mode=indexing
          i -> [w1035]
          n394 = Subtract(x=w1036, y=w1035) -> (x-y=w1034:dbl)
        }
        n395 = call "Wheel Pos Auto Adjust.vi"("Action"=enum16{"Initialize", "Analyzing", "Choosing"}."Initialize", "error in"=w1006) -> ("error out"=w1015:errorcluster)  [unwired: 5 in, 4 out]
        n396 = Number To Decimal String(number=w1028) -> (decimal integer string=w1023:string[])  [unwired: 1 in]
        n397 = call "SEQ Preview Queue.vi"("error in"=w1015) -> ("error out"=w1014:errorcluster, "SEQ Data"=w1012:T12)  [unwired: 9 in]
        n398 = Bundle By Name(cluster=w1012, "Align Done?"=FALSE) -> (w1011:T12)
        n399 = Array Size(array=w1023) -> (size(s)=w1022:i32)
        n400 = Format Date/Time String(time format string (%c)="%y%m%d_%H%M%S_") -> (date/time string=w1008:string)  [unwired: 2 in]
        n401 = Decrement(x=w1022) -> (x-1=w1021:i32)
        n402 = call "SEQ Lossy Queue.vi"("error in"=w1014, "SEQ Data"=w1011) -> ("error out"=w1013:errorcluster)  [unwired: 9 in]
        n403 = Bundle By Name(cluster=w1033, "Align Total"=w1021, "Align Count"=0 ("Acquire Count"), "Dichroic Position"=w1023, "Acquire Time"=w1008) -> (w1024:T5)
      }
      frame "Align Rotate 6" {
        n404 = call "Rotate U.vi"("Error In"=w1050, "Cube"=enum16{"1", "2", "3", "4", "5", "6", "7", "8"}."6") -> ("Error Out"=w1042:errorcluster)  [unwired: 9 in]
        n405 = call "Rendezvous Align.vi"("Error In"=w1042) -> ("Error Out"=w1041:errorcluster)  [unwired: 10 in]
        n406 = call <vilib>:"Create Rendezvous.vi"("error in (no error)"=w1041, "size (2)"=2, "name (unnamed)"="Align") -> ("error out"=w1049:errorcluster, "rendezvous"=w1046:T13)  [unwired: 2 in, 1 out]
        n407 = call <vilib>:"Wait at Rendezvous.vi"("error in (no error)"=w1049, "ms timeout (-1)"=10000, "rendezvous"=w1046) -> ("error out"=w1044:errorcluster, "timed out"=w1040:bool, "rendezvous out"=w1043:T13)  [unwired: 2 in]
        n408 = call <vilib>:"Destroy Rendezvous.vi"("error in (no error)"=w1044, "rendezvous"=w1043) -> ("error out"=w1039:errorcluster)  [unwired: 4 in, 1 out]
        n409 = case shown="False" w1040 {
          tunnel: w1039 -> [w1056 _]
          tunnel: w1038 -> [w1054 _]
          tunnel: [w1055 w1057] -> w1037
          frame False {
            n410 = call "Enqueue.vi"("Error In"=w1056, "State"="Align Rotate U", "Queue in"=w1054) -> ("Error Out"=w1055:errorcluster)  [unwired: 7 in, 1 out]
          }
          frame True {
            n411 = xnode "Error Ring"() -> ("error out"=w1057:errorcluster)
          }
        }
      }
      frame "Align Rotate U" {
        n412 = Unbundle By Name(w1066) -> ("Dichroic Position"=w1065:string[], "Align Count"=w1064:i32)
        n413 = Index Array(array=w1065, index=w1064) -> (element=w1063:string)
        n414 = call "Move Axis 4.vi"("Error In"=w1068, "Position"=w1063) -> ("Error Out"=w1067:errorcluster)  [unwired: 9 in]
        n415 = call "Rendezvous Align.vi"("Error In"=w1067) -> ("Error Out"=w1073:errorcluster)  [unwired: 10 in]
        n416 = call <vilib>:"Create Rendezvous.vi"("error in (no error)"=w1073, "size (2)"=2, "name (unnamed)"="Align") -> ("error out"=w1080:errorcluster, "rendezvous"=w1077:T13)  [unwired: 2 in, 1 out]
        n417 = call <vilib>:"Wait at Rendezvous.vi"("error in (no error)"=w1080, "ms timeout (-1)"=10000, "rendezvous"=w1077) -> ("error out"=w1075:errorcluster, "timed out"=w1072:bool, "rendezvous out"=w1074:T13)  [unwired: 2 in]
        n418 = call <vilib>:"Destroy Rendezvous.vi"("error in (no error)"=w1075, "rendezvous"=w1074) -> ("error out"=w1071:errorcluster)  [unwired: 4 in, 1 out]
        n419 = case shown="False" w1072 {
          tunnel: w1071 -> [w1082 _]
          tunnel: w1070 -> [w1084 _]
          tunnel: [w1085 w1088] -> w1069
          frame False {
            n420 = flat-sequence {
              tunnel: w1082 -> [w1087]
              tunnel: [w1087] -> w1081
              frame #0 {
                n421 = Wait (ms)(milliseconds to wait=u32 1000) -> ()  [unwired: 1 out]
              }
            }
            n422 = call "Enqueue.vi"("Error In"=w1081, "State"="Align Snap", "Queue in"=w1084) -> ("Error Out"=w1085:errorcluster)  [unwired: 7 in, 1 out]
          }
          frame True {
            n423 = xnode "Error Ring"() -> ("error out"=w1088:errorcluster)
          }
        }
      }
      frame "Align Snap" {
        n424 = call "Snap.vi"("Error In"=w1107) -> ("Error Out"=w1106:errorcluster)  [unwired: 10 in]
        n425 = call "Rendezvous Snap.vi"("Error In"=w1106) -> ("Error Out"=w1105:errorcluster)  [unwired: 10 in]
        n426 = call <vilib>:"Create Rendezvous.vi"("error in (no error)"=w1105, "size (2)"=2, "name (unnamed)"="Snap") -> ("error out"=w1104:errorcluster, "rendezvous"=w1102:T13)  [unwired: 2 in, 1 out]
        n427 = call <vilib>:"Wait at Rendezvous.vi"("error in (no error)"=w1104, "ms timeout (-1)"=5000, "rendezvous"=w1102) -> ("error out"=w1103:errorcluster, "timed out"=w1096:bool, "rendezvous out"=w1101:T13)  [unwired: 2 in]
        n428 = call <vilib>:"Destroy Rendezvous.vi"("error in (no error)"=w1103, "rendezvous"=w1101) -> ("error out"=w1097:errorcluster)  [unwired: 4 in, 1 out]
        n429 = case shown="False" w1096 {
          tunnel: w1097 -> [w1112 _]
          tunnel: [w1111 w1113] -> w1095
          tunnel: w1094 -> [w1110 _]
          frame False {
            n430 = call "Enqueue.vi"("Error In"=w1112, "State"="Align Analyze", "Queue in"=w1110) -> ("Error Out"=w1111:errorcluster)  [unwired: 7 in, 1 out]
          }
          frame True {
            n431 = xnode "Error Ring"() -> ("error out"=w1113:errorcluster)
          }
        }
      }
      frame "Align Analyze" {
        n432 = Unbundle By Name(w1127) -> ("Dichroic Position"=w1126:string[], "Align Count"=w1125:i32)
        n433 = call "SEQ Preview Queue.vi"("error in"=w1131) -> ("error out"=w1129:errorcluster, "SEQ Data"=w1130:T14)  [unwired: 9 in]
        n434 = Unbundle By Name(w1130) -> ("Image Ref"=w1128:T3)
        n435 = Index Array(array=w1126, index=w1125) -> (element=w1124:string)
        n436 = call "Wheel Pos Auto Adjust.vi"("Action"=enum16{"Initialize", "Analyzing", "Choosing"}."Analyzing", "error in"=w1129, "Wheel position"=w1124, "Refnum in"=w1128) -> ("error out"=w1122:errorcluster)  [unwired: 3 in, 4 out]
        n437 = call "Enqueue.vi"("Error In"=w1122, "State"="Align Next", "Queue in"=w1120) -> ("Error Out"=w1121:errorcluster)  [unwired: 7 in, 1 out]
      }
      frame "Align Next" {
        n438 = Unbundle By Name(w1140) -> ("Align Total"=w1139:i32, "Align Count"=w1137:i32)
        n439 = Equal?(x=w1139, y=w1137) -> (x = y?=w1138:bool)
        n440 = case shown="True" w1138 {
          tunnel: w1137 -> [w1146 _]
          tunnel: [w1145 0] -> w1132
          tunnel: w1136 -> [w1144 w1150]
          tunnel: w1135 -> [w1143 w1148]
          tunnel: [w1142 w1149] -> w1134
          frame False {
            n441 = Increment(x=w1146) -> (x+1=w1145:i32)
            n442 = call "Enqueue.vi"("Error In"=w1144, "State"="Align Rotate 6", "Queue in"=w1143) -> ("Error Out"=w1142:errorcluster)  [unwired: 7 in, 1 out]
          }
          frame True {
            n443 = call "Enqueue.vi"("Error In"=w1150, "State"="Align Choose", "Queue in"=w1148) -> ("Error Out"=w1149:errorcluster)  [unwired: 7 in, 1 out]
          }
        }
        n444 = Bundle By Name(cluster=w1140, "Align Count"=w1132) -> (w1133:T5)
      }
      frame "Align Choose" {
        n445 = call "Wheel Pos Auto Adjust.vi"("Action"=enum16{"Initialize", "Analyzing", "Choosing"}."Choosing", "error in"=w1159) -> ("error out"=w1157:errorcluster, "Best wheel position"=w1152:string, "No position match?"=w1156:bool)  [unwired: 5 in, 2 out]
        n446 = case shown="False" w1156 {
          selector: w1156 -> [w1165 w1175]
          tunnel: w1157 -> [w1170 w1179]
          tunnel: w1155 -> [w1162 w1172]
          tunnel: w1152 -> [w1166 _]
          tunnel: [w1163 w1173] -> w1154
          frame False {
            n447 = call "SEQ Preview Queue.vi"("error in"=w1170) -> ("error out"=w1169:errorcluster, "SEQ Data"=w1168:T12)  [unwired: 9 in]
            n448 = Bundle By Name(cluster=w1168, "No Position Match?"=w1165, "Best Wheel Position"=w1166) -> (w1167:T12)
            n449 = call "SEQ Lossy Queue.vi"("error in"=w1169, "SEQ Data"=w1167) -> ("error out"=w1164:errorcluster)  [unwired: 9 in]
            n450 = call "Enqueue.vi"("Error In"=w1164, "State"="Align Rotate 6 Final", "Queue in"=w1162) -> ("Error Out"=w1163:errorcluster)  [unwired: 7 in, 1 out]
          }
          frame True {
            n451 = call "SEQ Preview Queue.vi"("error in"=w1179) -> ("error out"=w1178:errorcluster, "SEQ Data"=w1177:T12)  [unwired: 9 in]
            n452 = Bundle By Name(cluster=w1177, "No Position Match?"=w1175) -> (w1176:T12)
            n453 = call "SEQ Lossy Queue.vi"("error in"=w1178, "SEQ Data"=w1176) -> ("error out"=w1174:errorcluster)  [unwired: 9 in]
            n454 = call "Enqueue.vi"("Error In"=w1174, "State"="Align End", "Queue in"=w1172) -> ("Error Out"=w1173:errorcluster)  [unwired: 7 in, 1 out]
          }
        }
        n455 = Bundle By Name(cluster=w1160, "Best Wheel Position"=w1152) -> (w1153:T5)
      }
      frame "Align Rotate 6 Final" {
        n456 = call "Rotate U.vi"("Error In"=w1193, "Cube"=enum16{"1", "2", "3", "4", "5", "6", "7", "8"}."6") -> ("Error Out"=w1185:errorcluster)  [unwired: 9 in]
        n457 = call "Rendezvous Align.vi"("Error In"=w1185) -> ("Error Out"=w1184:errorcluster)  [unwired: 10 in]
        n458 = call <vilib>:"Create Rendezvous.vi"("error in (no error)"=w1184, "size (2)"=2, "name (unnamed)"="Align") -> ("error out"=w1192:errorcluster, "rendezvous"=w1189:T13)  [unwired: 2 in, 1 out]
        n459 = call <vilib>:"Wait at Rendezvous.vi"("error in (no error)"=w1192, "ms timeout (-1)"=10000, "rendezvous"=w1189) -> ("error out"=w1187:errorcluster, "timed out"=w1183:bool, "rendezvous out"=w1186:T13)  [unwired: 2 in]
        n460 = call <vilib>:"Destroy Rendezvous.vi"("error in (no error)"=w1187, "rendezvous"=w1186) -> ("error out"=w1182:errorcluster)  [unwired: 4 in, 1 out]
        n461 = case shown="False" w1183 {
          tunnel: w1182 -> [w1199 _]
          tunnel: w1181 -> [w1197 _]
          tunnel: [w1198 w1200] -> w1180
          frame False {
            n462 = call "Enqueue.vi"("Error In"=w1199, "State"="Align Move to Best", "Queue in"=w1197) -> ("Error Out"=w1198:errorcluster)  [unwired: 7 in, 1 out]
          }
          frame True {
            n463 = xnode "Error Ring"() -> ("error out"=w1200:errorcluster)
          }
        }
      }
      frame "Align Move to Best" {
        n464 = Unbundle By Name(w1207) -> ("Best Wheel Position"=w1206:string)
        n465 = call "Move Axis 4.vi"("Error In"=w1209, "Position"=w1206) -> ("Error Out"=w1208:errorcluster)  [unwired: 9 in]
        n466 = call "Rendezvous Align.vi"("Error In"=w1208) -> ("Error Out"=w1214:errorcluster)  [unwired: 10 in]
        n467 = call <vilib>:"Create Rendezvous.vi"("error in (no error)"=w1214, "size (2)"=2, "name (unnamed)"="Align") -> ("error out"=w1221:errorcluster, "rendezvous"=w1218:T13)  [unwired: 2 in, 1 out]
        n468 = call <vilib>:"Wait at Rendezvous.vi"("error in (no error)"=w1221, "ms timeout (-1)"=10000, "rendezvous"=w1218) -> ("error out"=w1216:errorcluster, "timed out"=w1213:bool, "rendezvous out"=w1215:T13)  [unwired: 2 in]
        n469 = call <vilib>:"Destroy Rendezvous.vi"("error in (no error)"=w1216, "rendezvous"=w1215) -> ("error out"=w1212:errorcluster)  [unwired: 4 in, 1 out]
        n470 = case shown="False" w1213 {
          tunnel: w1212 -> [w1222 _]
          tunnel: w1211 -> [w1225 _]
          tunnel: [w1226 w1229] -> w1210
          frame False {
            n471 = flat-sequence {
              tunnel: [w1228] -> w1223
              tunnel: w1222 -> [w1228]
              frame #0 {
                n472 = Wait (ms)(milliseconds to wait=u32 1000) -> ()  [unwired: 1 out]
              }
            }
            n473 = call "Enqueue.vi"("Error In"=w1223, "State"="Align Snap Final", "Queue in"=w1225) -> ("Error Out"=w1226:errorcluster)  [unwired: 7 in, 1 out]
          }
          frame True {
            n474 = xnode "Error Ring"() -> ("error out"=w1229:errorcluster)
          }
        }
      }
      frame "Align Snap Final" {
        n475 = call "Snap.vi"("Error In"=w1248) -> ("Error Out"=w1247:errorcluster)  [unwired: 10 in]
        n476 = call "Rendezvous Snap.vi"("Error In"=w1247) -> ("Error Out"=w1246:errorcluster)  [unwired: 10 in]
        n477 = call <vilib>:"Create Rendezvous.vi"("error in (no error)"=w1246, "size (2)"=2, "name (unnamed)"="Snap") -> ("error out"=w1245:errorcluster, "rendezvous"=w1243:T13)  [unwired: 2 in, 1 out]
        n478 = call <vilib>:"Wait at Rendezvous.vi"("error in (no error)"=w1245, "ms timeout (-1)"=5000, "rendezvous"=w1243) -> ("error out"=w1244:errorcluster, "timed out"=w1237:bool, "rendezvous out"=w1242:T13)  [unwired: 2 in]
        n479 = call <vilib>:"Destroy Rendezvous.vi"("error in (no error)"=w1244, "rendezvous"=w1242) -> ("error out"=w1238:errorcluster)  [unwired: 4 in, 1 out]
        n480 = case shown="False" w1237 {
          tunnel: w1238 -> [w1253 _]
          tunnel: [w1252 w1254] -> w1236
          tunnel: w1235 -> [w1251 _]
          frame False {
            n481 = call "Enqueue.vi"("Error In"=w1253, "State"="Align Save", "Queue in"=w1251) -> ("Error Out"=w1252:errorcluster)  [unwired: 7 in, 1 out]
          }
          frame True {
            n482 = xnode "Error Ring"() -> ("error out"=w1254:errorcluster)
          }
        }
      }
      frame "Align Save" {
        n483 = Unbundle By Name(w1271) -> ("Image Path"=w1268:path, "Acquire Time"=w1270:string, "Best Wheel Position"=w1260:string)
        n484 = call "Enqueue.vi"("Error In"=w1264, "State"="Align End", "Queue in"=w1262) -> ("Error Out"=w1263:errorcluster)  [unwired: 7 in, 1 out]
        n485 = call "SEQ Preview Queue.vi"("error in"=w1263) -> ("error out"=w1273:errorcluster, "SEQ Data"=w1274:T14)  [unwired: 9 in]
        n486 = Concatenate Strings(w1270, w1260, ".tif" ("string")) -> (w1267:string)
        n487 = Unbundle By Name(w1274) -> ("Image Ref"=w1272:T3)
        n488 = Build Path(base path=w1268, name or relative path=w1267) -> (appended path=w1266:path)
        n489 = call-poly "IMAQ Write File 2"("error in (no error)"=w1273, "File Path"=w1266, "Image"=w1272) -> ("error out"=w1265:errorcluster)  [unwired: 7 in, 1 out]
      }
      frame "Align End" {
        n490 = call "Overlay Disable.vi"("Error In"=w1276) -> ("Error Out"=w1275:errorcluster)  [unwired: 10 in]
        n491 = call "Change Expo.vi"("Error In"=w1275, "Expo(s)"=0.05) -> ("Error Out"=w1279:errorcluster)  [unwired: 9 in]
        n492 = call "Grab.vi"("Error In"=w1279) -> ("Error Out"=w1278:errorcluster)  [unwired: 10 in]
        n493 = call "SEQ Preview Queue.vi"("error in"=w1278) -> ("error out"=w1284:errorcluster, "SEQ Data"=w1282:T12)  [unwired: 9 in]
        n494 = Bundle By Name(cluster=w1282, "Align Done?"=TRUE) -> (w1281:T12)
        n495 = call "SEQ Lossy Queue.vi"("error in"=w1284, "SEQ Data"=w1281) -> ("error out"=w1283:errorcluster)  [unwired: 9 in]
      }
      frame "------Error Handler------" {
      }
      frame "Error" {
        n496 = Variant To Data(error in=w1291, type=errorcluster {"status"=FALSE, "code"=0, "source"=""} ("error constant"), Variant=w1290) -> (data=w1292:errorcluster)  [unwired: 1 out]
        n497 = call <vilib>:"Simple Error Handler.vi"("error in (no error)"=w1292) -> ()  [unwired: 4 in, 5 out]
      }
      frame "------Close------" {
      }
      frame "Close" {
        n498 = for {
          tunnel: w1298 -> [w1302]
          shift-right: [w1303] -> w1297
          shift-left: w1299 -> [w1304]
          tunnel: string[] ["Release Queue"] -> [w1301] mode=indexing
          n499 = call "Enqueue.vi"("Error In"=w1304, "State"=w1301, "Queue in"=w1302) -> ("Error Out"=w1303:errorcluster)  [unwired: 7 in, 1 out]
        }
      }
      frame "Release Queue" {
        n500 = Release Queue(queue=w1314, error in (no error)=w1315) -> (error out=w1313:errorcluster)  [unwired: 1 in, 2 out]
        n501 = call "SEQ Release Queue.vi"("error in"=w1313) -> ("error out"=w1312:errorcluster)  [unwired: 10 in]
        n502 = Unbundle By Name(w1311) -> ("Temp Image(U8)"=w1305:T3, "Pattern Image(U8)"=w1306:T3, "Temp Image(U16)"=w1310:T3)
        n503 = call "IMAQ Dispose"("Image"=w1310, "error in (no error)"=w1312) -> ("error out"=w1309:errorcluster)  [unwired: 4 in]
        n504 = call "IMAQ Dispose"("Image"=w1306, "error in (no error)"=w1309) -> ("error out"=w1308:errorcluster)  [unwired: 4 in]
        n505 = call "IMAQ Dispose"("Image"=w1305, "error in (no error)"=w1308) -> ("error out"=w1307:errorcluster)  [unwired: 4 in]
      }
    }
    n506 = case shown="Error .." w137 {
      selector: w137 -> [w1317 w1321]
      tunnel: [w1317 w1322] -> w138
      tunnel: w136 -> [_ w1319]
      frame No Error {
      }
      frame Error {
        n507 = To Variant(anything=w1321) -> (Variant=w1320:variant)
        n508 = call "Enqueue.vi"("Data"=w1320, "State"="Error", "Queue in"=w1319) -> ("Error Out"=w1322:errorcluster)  [unwired: 7 in, 1 out]
      }
    }
  }
  n509 = Merge Errors(w8, w6) -> (→"error out":errorcluster)
